vi "Multi_Run_Prog.vi"(0 "Command filename":path, 1 "Mode":T9(ring), 2 "Table":T6[](array[typedef]) {"Carrier_2 Q (l/min)" format="%#.2f"; "Row Duration (mins)" format="%#.1f"; "Row No" min=0; "Trace Gas Concentration (%)" min=0.0 format="%#_4f"; "Carrier_1 Q (l/min)" format="%#.2f"; "Tunnel Speed" format="%#.2f"; "Start X" format="%#.2f"; "Start Y" format="%#.2f"; "Start Z" format="%#.2f"; "End X" format="%#.2f"; "End Y" format="%#.2f"; "End Z" format="%#.2f"; "Averaging time (min)" min=0.0 format="%#.2f"}, 3 "Work in Tunnel Coordinates?":T1, 4 "Jump Bad Positions":bool) -> ()   [LabVIEW 2015]
uses:
  Anemometry Sub Vis/Gen Trav/Traverse_cluster.ctl
  Anemometry Sub Vis/Gen Trav/Spacing.ctl
  Anemometry Sub Vis/Controls/Multi_run_mode.ctl
  Anemometry Sub Vis/Gen Trav/Route mapping/Route_Display_Mode.ctl
  Anemometry Sub Vis/Controls/User_Specific_mode.ctl
  Anemometry Sub Vis/Controls/Multi_Run_Case.ctl
  Anemometry Sub Vis/Gen Trav/Multi_Run_Status.ctl
  Anemometry Sub Vis/Controls/Tunnel_Coordinates.ctl
  Anemometry Sub Vis/Controls/Post_Process.ctl
  ADAM Client/Sub VIs/ADAM Controls/Traverse_Level_State.ctl
  ADAM Client/Sub VIs/ADAM Controls/Tunnel_speed_mode.ctl
  Anemometry Sub Vis/Controls/Overhead.ctl
  ADAM Client/Sub VIs/ADAM Controls/Remember_value_mode.ctl
  Anemometry Sub Vis/Gen Trav/Trav_mode.ctl
  Anemometry Sub Vis/Controls/Home.ctl
  ADAM Client/Sub VIs/ADAM Controls/Client_Source_Status.ctl
  ADAM Client/Sub VIs/ADAM Controls/Update_scan_value.ctl
  Anemometry Sub Vis/File/Setup_Filetype.ctl
  Anemometry Sub Vis/Globals/Meas_global.vi
  Anemometry Sub Vis/Globals/Trav_pos_global.vi
  Anemometry Sub Vis/Globals/Preference_global.vi
  Anemometry Sub Vis/Gen Trav/Route mapping/Route_mapping_global.vi
  ADAM Serial/Instrument drivers/Traverses/~subVIs/DriveConfigGlobal.vi
  Anemometry Sub Vis/Globals/Extra_Commands_Global.vi
panel:
  in  "Sort Single\nMeasurements":bool
  out "Last Row Run":i32
  in  "Stop after Repeats":bool
  out "Current Overhead Factor":dbl format="%.3f"
  out "Estimated Completion time":string
  out "Max Tunnel Speed":dbl format="%.2f"
  out "Pause message":string
  in  "Pause":bool
  out "Non Starter":bool
  out "No of Rows":i32
  out "Status":T2
  in  "Synchronization Start No":i32=1 min=1 max=100
  out "Multi Run Case":T3
  out "Simulate/Run":T4
  in  "Display Mode":T5=enum."Display View on Crash"
  in  "stop":bool
  out "Currently on Row":i32
  # "X           Y            Z"
  # "Start"
  # "End"
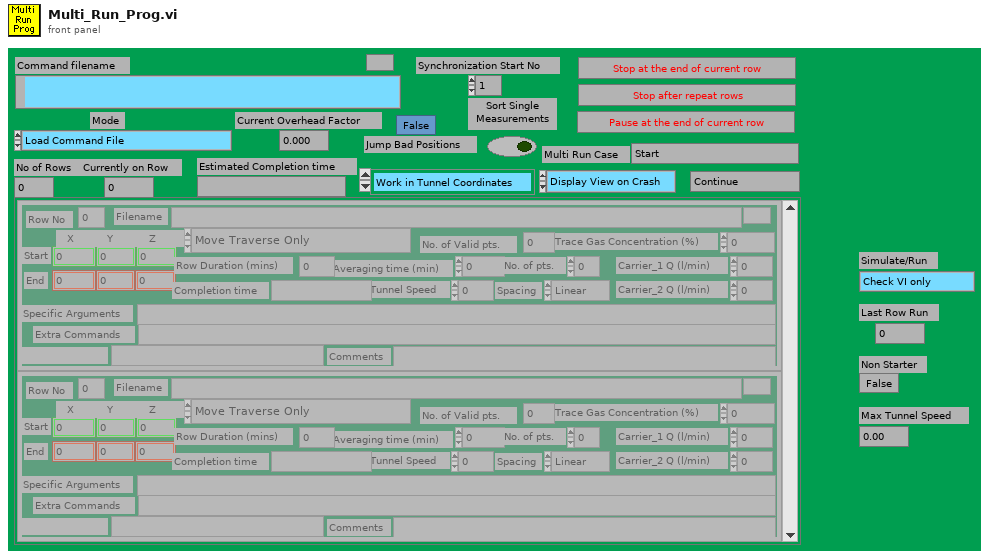
[diagram p1: front panel]
types:
  T1 = typedef "Tunnel_Coordinates.ctl" = enum16{"Work in Tunnel Coordinates", "Work in Model Coordinates"}
  T2 = typedef "Multi_Run_Status.ctl" = enum16{"Continue", "Jump to Next Point", "Jump to Next Row", "Jump To Fall Back", "Terminate Run"}
  T3 = typedef "Multi_Run_Case.ctl" = enum16{"Start", "Load Setup From File", "Has file been edited in Excel?", "Check Max Tunnel Speed", "Pre Check Row", "Check Rows", "Remove blank end rows", "Do results files already exist?", "FFID Bkgnd Measurements?", "First Save Setup file", "Setup Route checking", "Initialise Measurement Prog", "Input Current Position", "Experimental setup control", "Check source flowrates", "Setup for running mode", "Skip Blank Rows", "Which row to execute next", "Evaluate IF Statement", "Perform Measurement Setup", "Set Measurement Conditions", "Execute Row", "Calculate Row TIme", "Update time estimate", "Pause Multi Run Program", "Do Another Row?", "Find Next Fall Back Row", "Shut down source etc", "Email results to users", "Save run efficiency", "Remove Skipped Commands", "Show jumped positions", "Save Setup to File", "End"}
  T4 = typedef "User_Specific_mode.ctl" = enum16{"Check VI only", "Run VI"}
  T5 = typedef "Route_Display_Mode.ctl" = enum16{"Display View Always", "Display View on Crash"}
  T6 = typedef "Traverse_cluster.ctl" = cluster{"Start X":sgl, "Start Y":sgl, "Start Z":sgl, "End X":sgl, "End Y":sgl, "End Z":sgl, "No. of pts.":i32, "Spacing":T7, "Filename":path, "Tunnel Speed":dbl, "Averaging time (min)":dbl, "Extra Commands":string, "Carrier_1 Q (l/min)":dbl, "Carrier_2 Q (l/min)":dbl, "Trace Gas Concentration (%)":dbl, "Specific Arguments":string, "Comments":string, "Row No":i32, "Row Type Selector":T8, "Completion time":string, "Row Duration (mins)":dbl, "No. of Valid pts.":i32, "Meas Setup File":string}
  T7 = typedef "Spacing.ctl" = enum16{"Linear", "Log", "Gauss", "Specified", "N/A"}
  T8 = typedef "Multi_run_mode.ctl" = enum16{"Move Traverse Only", "Set Tunnel Speed Only", "Set Source Only", "Set Measurement Conditions", "Single Measurement", "Vertical Profile", "Lateral Profile", "Longitudinal Profile", "Explore Volume", "Multi-Axis Profile", "Auto Calibrate", "Meas Fast FID Bkgnd", "Check Beam Power", "Scanning Valve Measurement", "Run VI Named:", "Set ADAM Ch", "Wait (minutes)", "Send Message", "Synchronize With:", "Fall Back to this Row", "Turn Off Row Repeating", "Blank Row", "Traverse 3D Volume"}
  T9 = enum16{"Load Command File", "Save Command File", "Check Multi Run Prog", "Check Multi Run Prog With Live Moves", "Run Multi Run Prog"}
  T10 = typedef "Post_Process.ctl" = enum16{"Take New Data", "Post Process Raw Data File"}
  T11 = typedef "Traverse_Level_State.ctl" = enum16{"Running", "Complete"}
  T12 = enum32{"existing file", "new file", "new or existing file", "existing dir", "new dir", "new or existing dir", "existing file (use LLBs)", "new file (use LLBs)", "new or existing file (use LLBs)", "new or existing file or directory (use LLBs)"}
  T13 = typedef "Tunnel_speed_mode.ctl" = enum16{"Set Speed", "Set Speed then wait", "Is tunnel speed allowable?"}
  T14 = enum16{"All Channel Names", "Valid Channel Names"}
  T15 = typedef "Overhead.ctl" = enum16{"Update total times", "Read Current Overhead", "Re Scale totals to 3 hrs", "Initialise totals to 3hr"}
  T16 = typedef "Remember_value_mode.ctl" = enum16{"Read only", "Read and Write"}
  T17 = typedef "Home.ctl" = enum16{"Don't Home", "Home  +X", "Home  -X", "Home  +Y", "Home  -Y", "Home  +Z", "Home  -Z"}
  T18 = typedef "Trav_mode.ctl" = enum16{"Move traverse", "Read traverse position", "Teach Position"}
  T19 = typedef "Client_Source_Status.ctl" = enum16{"Not Using", "Using", "Must Have"}
  T20 = typedef "Update_scan_value.ctl" = cluster{"Channel Name":string, "New Value":dbl}
  T21 = typedef "Setup_Filetype.ctl" = enum16{"Measurement Setups", "Calibration Setups", "General", "Results File Plotter Setups", "Speed Calib Tweaks"}
  T22 = typedef "AxisConfigCluster.ctl" = cluster{"Channel Properties":T23, "Static Drive Configuration":T24}
  T23 = typedef "DriveProperties.ctl" = cluster{"Channel Name":string, "Vel. Default":sgl, "Acc. Default":sgl, "Vel. Max":sgl, "Vel. Min":sgl, "Acc. Max":sgl, "Acc. Min":sgl, "Pulses/unit":sgl, "Address":u8, "Pulse Offset":i32, "Pos Tolerance":sgl, "Pulses/rev":sgl, "Backlash/Eng units":sgl, "Current Pos":sgl, "Ch Status":enum16{"Active", "Offline", "Simulate"}, "Port Name":string, "Axis Transform mode":string, "Metadata Ch Name":string, "Type":string}
  T24 = typedef "DriveStaticConfig.ctl" = cluster{"Correction Gain % (CG)":u16, "Dead Band (DB)":i32, "Dead Band Window (DW)":i32, "Encoder Resolution (ER)":i32, "Step Mode  (FSB)":u16, "Position Maintenance (FSC)":u16, "Stop on Stall (FSD)":u16, "Activate OP1 on stall (FSE)":u16, "Stop on Trigger 3 (FSF)":u16, "OP2 in Deadband (FSG)":u16, "Stall Detect (FSH)":u16, "Limit Disable (LD)":u16, "Motor Resolution (MR)":enum16{"200", "400", "1000", "2000", "4000", "5000", "10000", "12800", "18000", "20000", "21600", "25000", "25400", "25600", "36000", "50000", "278528", "425984", "507904", "614400", "655360", "819200", "1024000"}, "Limit Switch Sense (OSA)":u16, "Home Position (OSB)":u16, "Home Switch Sense (OSC)":u16, "Encoder Z for Home (OSD)":u16, "Reference edge of Home (OSH)":u16, "RS232 Echo Control (SSA)":u16, "Buffer at Limit (SSG)":u16, "Buffer at Stop (SSH)":u16, "Indexer Mode  (FSA)":u16, "Type":string, "ConfigString":string, "De Power Motor":enum16{"TRUE", "FALSE"}}
  T25 = typedef "Status_Cluster.ctl" = cluster{"Status":T2, "Error Type":string, "Error Description":string}
  T26 = typedef "Server_Comms.ctl" = enum16{"Server Link Healthy", "Do Not Link To Server"}
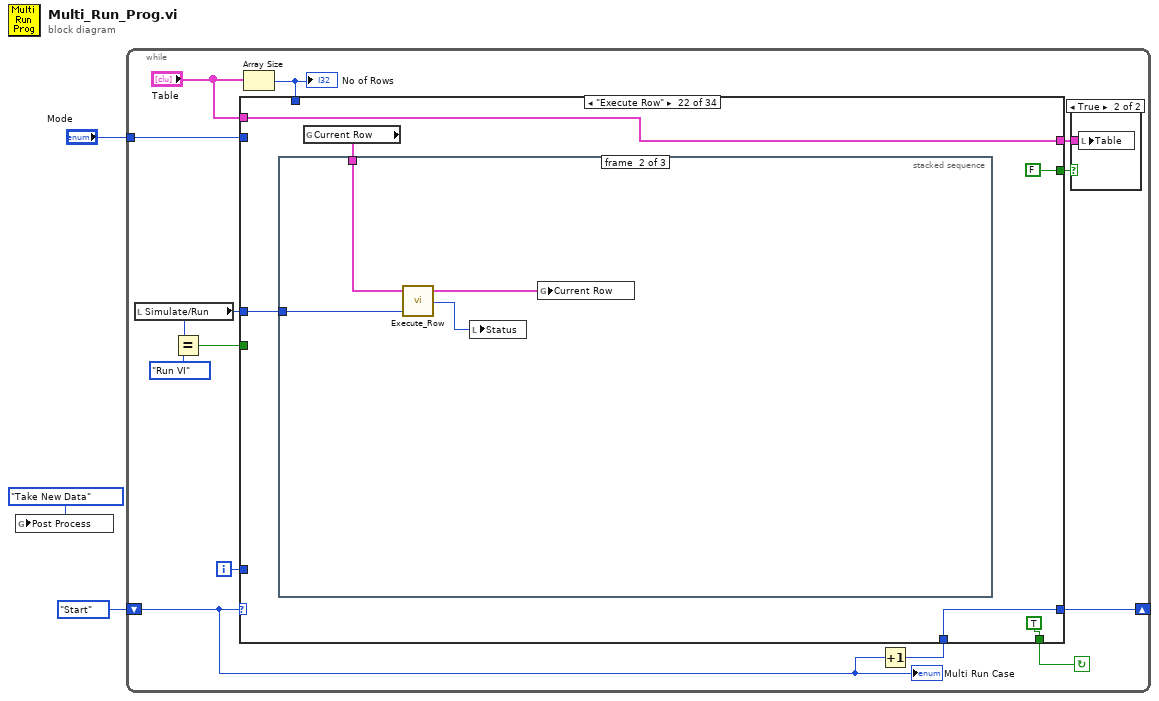
[diagram p0: block diagram]
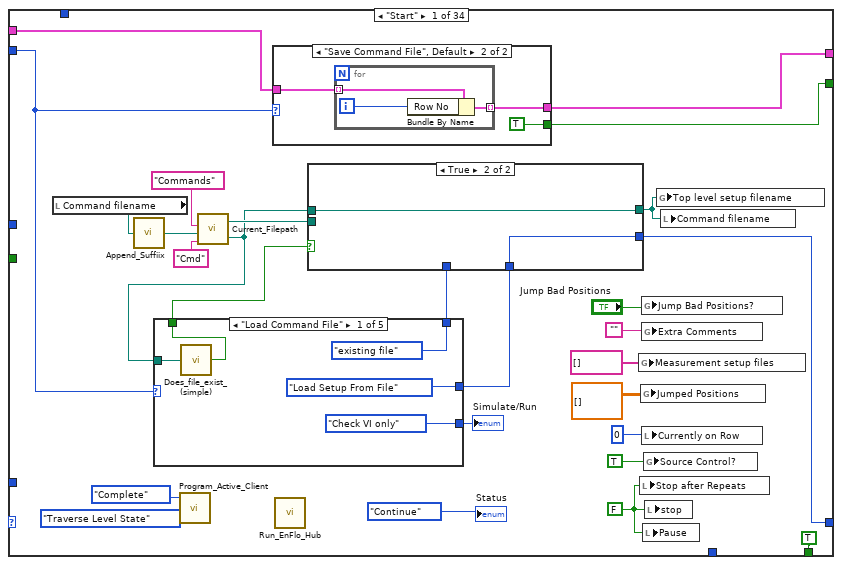
[diagram p3: hidden frame]
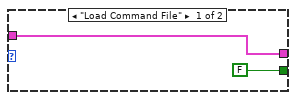
[diagram p4: hidden frame]
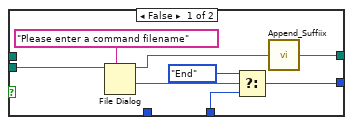
[diagram p5: hidden frame]
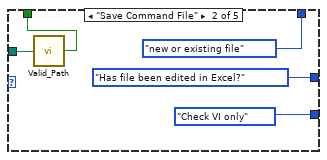
[diagram p6: hidden frame]
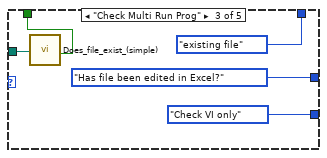
[diagram p7: hidden frame]
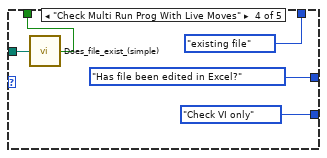
[diagram p8: hidden frame]
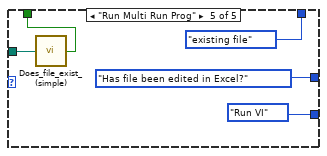
[diagram p9: hidden frame]
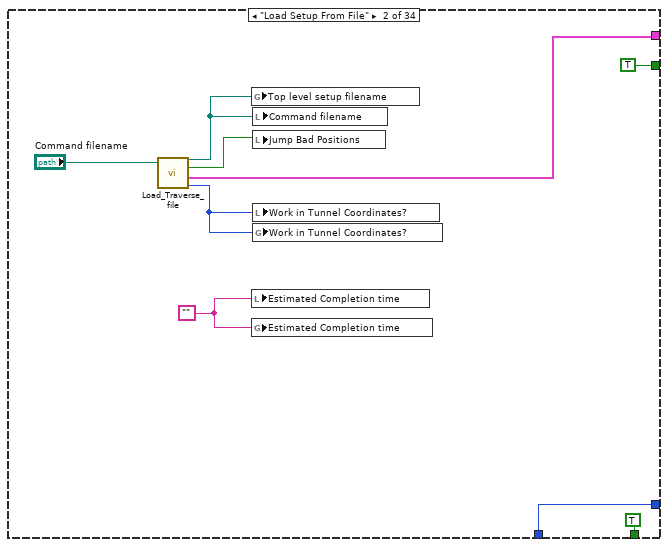
[diagram p10: hidden frame]
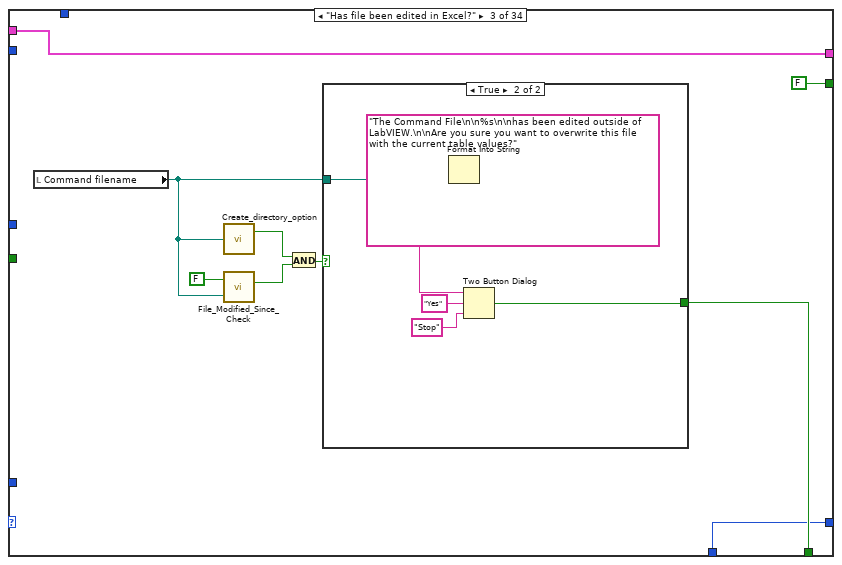
[diagram p11: hidden frame]
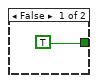
[diagram p12: hidden frame]
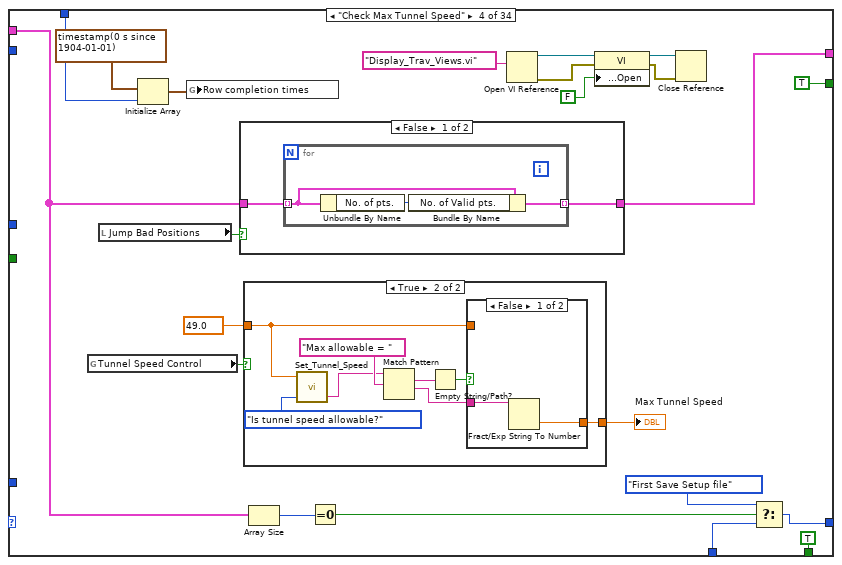
[diagram p13: hidden frame]
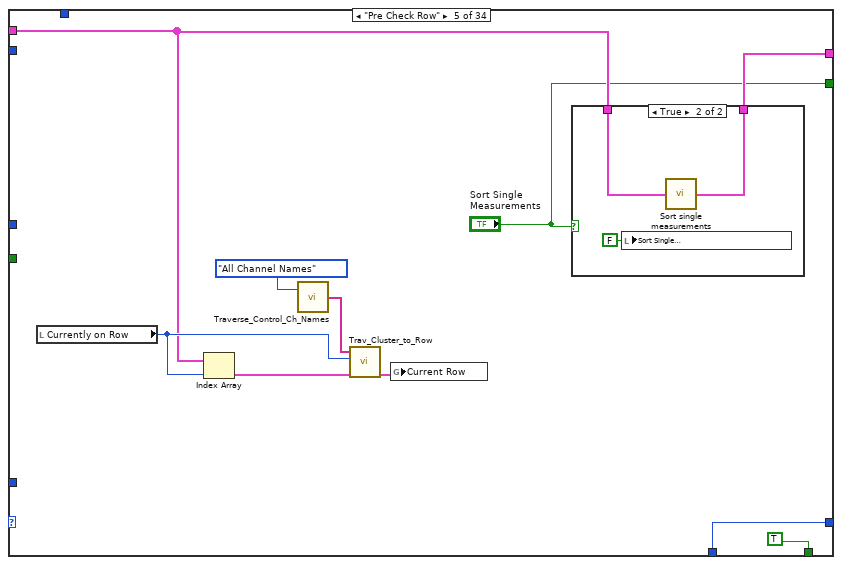
[diagram p17: hidden frame]
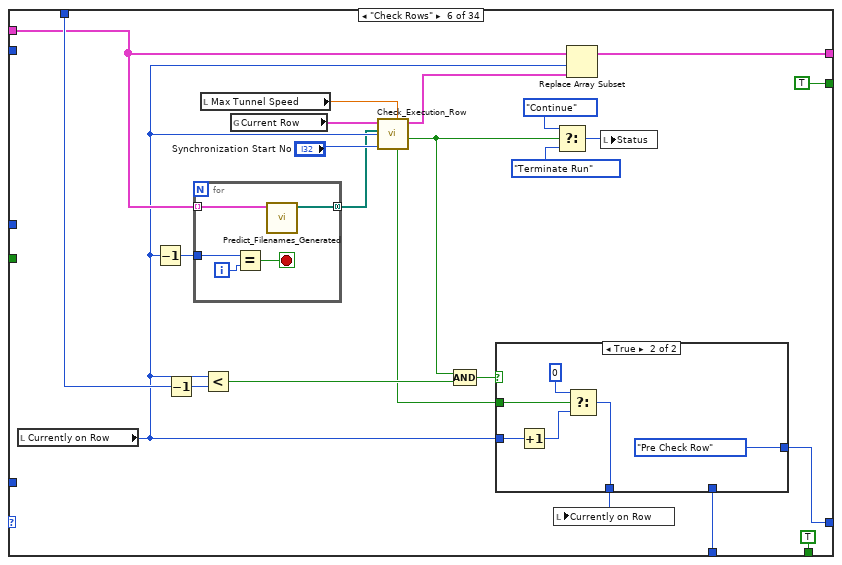
[diagram p19: hidden frame]
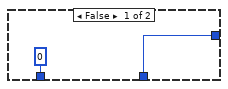
[diagram p20: hidden frame]
diagram:
  n1 = global write "Meas_global.vi" "Post Process"(Post_Process."Take New Data" ("Post Process")) -> ()
  n2 = while {
    shift-left: Multi_Run_Case."Start" ("Multi Run Case") -> [w12]
    shift-right: [w9] -> _
    tunnel: "Mode" -> [w15]
    i -> [w13]
    stop <- w16 continue-if-true
    n3 = local read "Simulate/Run"() -> (w5:T4)
    n4 = Equal?(x=w5, y=User_Specific_mode."Run VI" ("Simulate/Run")) -> (x = y?=w4:bool)
    n5 = Array Size(array="Table") -> (size(s)=w8:i32)
    "No of Rows" <- w8
    n6 = Increment(x=w12) -> (x+1=w14:T3)
    n7 = case shown="\"Execute Row\"" w12 {
      tunnel: [TRUE TRUE w100 TRUE TRUE TRUE TRUE TRUE TRUE TRUE TRUE ("Continue?") TRUE ("Continue?") TRUE TRUE TRUE w544 TRUE ("Continue?") TRUE ("Continue?") TRUE TRUE ("Continue?") TRUE TRUE TRUE TRUE TRUE TRUE TRUE TRUE TRUE TRUE TRUE TRUE TRUE FALSE] -> w16
      tunnel: w15 -> [w30 _ _ _ _ _ _ _ _ w426 _ _ _ _ _ _ _ _ _ _ _ _ _ _ _ _ _ _ _ _ _ _ w1267 _]
      tunnel: "Table" -> [w42 _ w97 w127 w155 w170 w204 w235 w393 w428 w451 w506 w518 w525 w533 w547 w609 w653 w757 w808 w820 w910 w944 w976 w1019 w1063 w1108 w1137 w1162 w1209 w1214 w1223 w1286 w1349]
      tunnel: w5 -> [_ _ _ _ _ _ _ w234 _ _ _ _ _ _ w532 w546 _ w651 _ w805 w817 w909 _ w973 _ w1069 _ _ _ _ _ _ w1277 _]
      tunnel: w14 -> [_ w93 w99 w125 w161 w176 w215 w238 w390 w425 w454 w504 w519 w524 w537 w549 w611 w649 w762 w809 w827 w907 w937 w978 w1022 _ _ w1123 w1164 w1211 w1217 w1231 w1284 w1348]
      tunnel: w13 -> [_ _ _ _ _ _ _ _ _ _ _ _ _ _ _ _ _ _ _ _ _ _ _ _ w1020 _ _ _ _ _ _ _ _ _]
      tunnel: [w40 w93 w99 w124 w161 w175 w215 w238 w390 w421 w454 w503 w519 w524 w535 w549 w611 w650 w761 w809 w828 w907 w937 w978 w1023 w1058 w1106 w1132 w1164 w1211 w1217 w1231 w1284 w1348] -> w9
      tunnel: [w29 TRUE FALSE ("Rows Added ?") TRUE ("Rows Added ?") "Sort Single\nMeasurements" TRUE TRUE FALSE FALSE TRUE FALSE FALSE FALSE FALSE FALSE TRUE FALSE ("Rows Added ?") FALSE ("Rows Added ?") FALSE FALSE ("Rows Added ?") FALSE FALSE FALSE TRUE ("Rows Added ?") FALSE FALSE FALSE FALSE FALSE FALSE TRUE TRUE TRUE FALSE] -> w10
      tunnel: w8 -> [_ _ _ w119 _ w180 w206 _ _ _ _ _ _ _ _ _ w612 w652 _ _ _ _ _ w972 _ w1061 w1099 _ _ _ _ _ w1258 _]
      tunnel: [w41 w94 w97 w129 w154 w183 w210 w235 w393 w429 w451 w506 w518 w525 w533 w545 w609 w654 w757 w808 w820 w910 w944 w975 w1019 w1063 w1108 w1137 w1162 w1209 w1213 w1223 w1285 w1349] -> w7
      tunnel: w4 -> [_ _ _ _ _ _ _ _ _ _ _ _ _ w522 w531 _ _ _ w751 _ _ _ w936 _ _ _ _ _ _ _ _ _ _ _]
      frame "Start" {
        w27 = FALSE ("Measurment setup Found?")
        n8 = local read "Command filename"() -> (w32:path)
        n9 = call "Append_Suffiix.vi"("Results file"=w32) -> ("appended path"=w22:path)
        n10 = call "Program_Active_Client.vi"("Mode"=enum16{"Program Active", "Traverse Level State"}."Traverse Level State", "Traverse level State"=Traverse_Level_State."Complete") -> ()  [unwired: 1 in, 3 out]
        n11 = call "Current_Filepath.vi"("Short_Name"="Cmd" ("Data Type"), "Filename in"=w22, "Data Type"="Commands") -> ("Filename Out"=w19:path, "Directory"=w21:path)  [unwired: 1 in]
        n12 = case shown="\"Load Command File\"" w30 {
          tunnel: [User_Specific_mode."Check VI only" ("Simulate/Run") User_Specific_mode."Check VI only" ("Simulate/Run") User_Specific_mode."Check VI only" ("Simulate/Run") User_Specific_mode."Check VI only" ("Simulate/Run") User_Specific_mode."Run VI" ("Simulate/Run")] -> w43
          tunnel: [Multi_Run_Case."Load Setup From File" ("Multi Run Case") Multi_Run_Case."Has file been edited in Excel?" ("Multi Run Case") Multi_Run_Case."Has file been edited in Excel?" ("Multi Run Case") Multi_Run_Case."Has file been edited in Excel?" ("Multi Run Case") Multi_Run_Case."Has file been edited in Excel?" ("Multi Run Case")] -> w39
          tunnel: [T12."existing file" ("select mode (2)") T12."new or existing file" ("select mode (2)") T12."existing file" ("select mode (2)") T12."existing file" ("select mode (2)") T12."existing file" ("select mode (2)")] -> w28
          tunnel: w19 -> [w64 w69 w73 w79 w84]
          tunnel: [w63 w68 w74 w78 w83] -> w18
          frame "Load Command File" {
            n13 = call "Does_file_exist_(simple).vi"("Pathname"=w64) -> ("exists?"=w63:bool)
          }
          frame "Save Command File" {
            n14 = call "Valid_Path.vi"("Filename"=w69) -> ("Valid Path?"=w68:bool)
          }
          frame "Check Multi Run Prog" {
            n15 = call "Does_file_exist_(simple).vi"("Pathname"=w73) -> ("exists?"=w74:bool)
          }
          frame "Check Multi Run Prog With Live Moves" {
            n16 = call "Does_file_exist_(simple).vi"("Pathname"=w79) -> ("exists?"=w78:bool)
          }
          frame "Run Multi Run Prog" {
            n17 = call "Does_file_exist_(simple).vi"("Pathname"=w84) -> ("exists?"=w83:bool)
          }
        }
        "Simulate/Run" <- w43
        n18 = case shown="\"Save Command File\", Default" w30 {
          tunnel: w42 -> [w46 w49]
          tunnel: [w46 w48] -> w41
          tunnel: [FALSE TRUE] -> w29
          frame "Load Command File" {
          }
          frame "Save Command File", Default {
            n19 = for {
              tunnel: w49 -> [w52] mode=indexing
              tunnel: [w51] -> w48 mode=indexing
              i -> [w50]
              n20 = Bundle By Name(cluster=w52, "Row No"=w50) -> (w51:T6)
            }
          }
        }
        n21 = call "Run_EnFlo_Hub.vi"() -> ()  [unwired: 8 out]
        n22 = case shown="True" w18 {
          tunnel: [w58 w62] -> w40
          tunnel: w39 -> [w59 w62]
          tunnel: w19 -> [_ w61]
          tunnel: [w57 w61] -> w31
          tunnel: w28 -> [_ _]
          tunnel: w21 -> [w53 _]
          frame False {
            n23 = File Dialog(7:"Please enter a command filename" ("prompt"), 11:w53) -> (1:w55:bool, 3:w56:path)  [unwired: 1 in, 6 out]
            n24 = Select(t=Multi_Run_Case."End" ("Multi Run Case"), s=w55, f=w59) -> (s? t:f=w58:T3)
            n25 = call "Append_Suffiix.vi"("Results file"=w56) -> ("appended path"=w57:path)
          }
          frame True {
          }
        }
        n26 = global write "Trav_pos_global.vi" "Measurement setup files"(string[] [] ("Measurement setup files")) -> ()
        n27 = local write "Stop after Repeats"(w27) -> ()
        n28 = global write "Trav_pos_global.vi" "Jumped Positions"(dbl[][] [] ("Jumped Positions")) -> ()
        n29 = global write "Trav_pos_global.vi" "Jump Bad Positions?"("Jump Bad Positions") -> ()
        n30 = global write "Meas_global.vi" "Extra Comments"("") -> ()
        n31 = local write "Currently on Row"(0 ("Currently on Row")) -> ()
        n32 = local write "Pause"(w27) -> ()
        n33 = global write "Trav_pos_global.vi" "Source Control?"(TRUE ("Source Control?")) -> ()
        n34 = local write "stop"(w27) -> ()
        n35 = global write "Trav_pos_global.vi" "Top level setup filename"(w31) -> ()
        n36 = local write "Command filename"(w31) -> ()
        "Status" <- Multi_Run_Status."Continue" ("Status")
      }
      frame "Load Setup From File" {
        w89 = ""
        n37 = call "Load_Traverse_file.vi"("Setup filename"="Command filename") -> ("Setup filename Out"=w91:path, "Jump Bad Positions"=w88:bool, "Table"=w94:T6[], "Work in Tunnel Coordinates?"=w90:T1)  [unwired: 2 out]
        n38 = global write "Trav_pos_global.vi" "Top level setup filename"(w91) -> ()
        n39 = local write "Estimated Completion time"(w89) -> ()
        n40 = global write "Trav_pos_global.vi" "Estimated Completion time"(w89) -> ()
        n41 = local write "Command filename"(w91) -> ()
        n42 = local write "Jump Bad Positions"(w88) -> ()
        n43 = local write "Work in Tunnel Coordinates?"(w90) -> ()
        n44 = global write "Trav_pos_global.vi" "Work in Tunnel Coordinates?"(w90) -> ()
      }
      frame "Has file been edited in Excel?" {
        n45 = local read "Command filename"() -> (w101:path)
        n46 = call "Create_directory_option.vi"("Filename"=w101) -> ("Path is to existing File"=w104:bool)  [unwired: 1 out]
        n47 = call "File_Modified_Since_Check.vi"("Pathname"=w101, "Just Modified?"=FALSE) -> ("Modified?"=w103:bool)
        n48 = And(x=w104, y=w103) -> (x .and. y?=w105:bool)
        n49 = case shown="True" w105 {
          tunnel: w101 -> [_ w112]
          tunnel: [TRUE ("T button?") w107] -> w100
          frame False {
          }
          frame True {
            n50 = Format Into String(format string="The Command File\n\n%s\n\nhas been edited outside of LabVIEW.\n\nAre you sure you want to overwrite this file  with the current table values?" ("Format String"), w112) -> (resulting string=w110:string)  [unwired: 2 in, 1 out]
            n51 = Two Button Dialog(message=w110, 1:"Stop" ("F button name (\"Cancel\")"), 2:"Yes" ("T button name (\"OK\")")) -> (T button?=w107:bool)
          }
        }
      }
      frame "Check Max Tunnel Speed" {
        n52 = global read "Preference_global.vi" "Tunnel Speed Control"() -> (w130:bool)
        n53 = local read "Jump Bad Positions"() -> (w128:bool)
        n54 = Initialize Array(timestamp(0 s since 1904-01-01) ("seconds since 1Jan1904"), w119) -> (w120:timestamp[])
        n55 = global write "Trav_pos_global.vi" "Row completion times"(w120) -> ()
        n56 = case shown="False" w128 {
          tunnel: w127 -> [w136 w140]
          tunnel: [w135 w140] -> w129
          frame False {
            n57 = for {
              tunnel: w136 -> [w138] mode=indexing
              tunnel: [w137] -> w135 mode=indexing
              n58 = Unbundle By Name(w138) -> ("No. of pts."=w139:i32)
              n59 = Bundle By Name(cluster=w138, "No. of Valid pts."=w139) -> (w137:T6)
            }
          }
          frame True {
          }
        }
        n60 = case shown="True" w130 {
          tunnel: 49.0 ("Tunnel Velocity m/s") -> [w141 w142]
          tunnel: [w141 w144] -> w132
          frame False {
          }
          frame True {
            n61 = call "Set_Tunnel_Speed.vi"("Mode"=Tunnel_speed_mode."Is tunnel speed allowable?", "Tunnel Velocity m/s"=w142) -> ("Error String"=w147:string)  [unwired: 1 in, 2 out]
            n62 = Match Pattern(string=w147, regular expression="Max allowable = ") -> (match substring=w146:string, after substring=w143:string)  [unwired: 3 out]
            n63 = Empty String/Path?(string/path=w146) -> (empty?=w145:bool)
            n64 = case shown="False" w145 {
              tunnel: [w150 w152] -> w144
              tunnel: w142 -> [_ w152]
              tunnel: w143 -> [w151 _]
              frame False {
                n65 = Fract/Exp String To Number(string=w151) -> (number=w150:dbl)  [unwired: 4 out]
              }
              frame True {
              }
            }
          }
        }
        "Max Tunnel Speed" <- w132
        n66 = Array Size(array=w127) -> (size(s)=w126:i32)
        n67 = Equal To 0?(x=w126) -> (x = 0?=w123:bool)
        n68 = Open VI Reference(vi path="Display_Trav_Views.vi" ("VI path")) -> (vi reference=w118:refnum<vi>, error out=w117:errorcluster)  [unwired: 1 in, 4 out]
        n69 = property class="VI"(reference=w118, error in=w117, "Front Panel Window:Open"=FALSE) -> (reference out=w115:refnum<vi>, error out=w114:errorcluster)
        n70 = Close Reference(reference=w115, error in (no error)=w114) -> ()  [unwired: 1 out]
        n71 = Select(t=Multi_Run_Case."First Save Setup file" ("Multi Run Case"), s=w123, f=w125) -> (s? t:f=w124:T3)
      }
      frame "Pre Check Row" {
        n72 = local read "Currently on Row"() -> (w158:i32)
        n73 = Index Array(array=w155, index=w158) -> (element=w159:T6)
        n74 = call "Traverse_Control_Ch_Names.vi"("Mode"=T14."All Channel Names") -> ("Channel names"=w156:string[])  [unwired: 1 in]
        n75 = call "Trav_Cluster_to_Row.vi"("Traverse line in"=w159, "Row Number"=w158, "Channel names"=w156) -> ("Traverse line Out"=w160:T6)  [unwired: 4 out]
        n76 = global write "Trav_pos_global.vi" "Current Row"(w160) -> ()
        n77 = case shown="True" "Sort Single\nMeasurements" {
          tunnel: w155 -> [w163 w166]
          tunnel: [w163 w165] -> w154
          frame False {
          }
          frame True {
            n78 = local write "Sort Single\nMeasurements"(FALSE ("Sort Single\nMeasurements")) -> ()
            n79 = call "Sort single measurements.vi"("Table In"=w166) -> ("Table Out"=w165:T6[])
          }
        }
      }
      frame "Check Rows" {
        n80 = local read "Currently on Row"() -> (w169:i32)
        n81 = Decrement(x=w169) -> (x-1=w168:i32)
        n82 = Decrement(x=w180) -> (x-1=w173:i32)
        n83 = for {
          tunnel: w170 -> [w194] mode=indexing
          tunnel: w168 -> [w192]
          tunnel: [w190] -> w167 mode=concatenating
          i -> [w193]
          stop <- w191 stop-if-true
          n84 = Equal?(x=w192, y=w193) -> (x = y?=w191:bool)
          n85 = call "Predict_Filenames_Generated.vi"("Traverse line"=w194) -> ("Filename"=w190:path[])  [unwired: 10 in]
        }
        n86 = local read "Max Tunnel Speed"() -> (w182:dbl)
        n87 = Less?(x=w169, y=w173) -> (x < y?=w179:bool)
        n88 = global read "Trav_pos_global.vi" "Current Row"() -> (w171:T6)
        n89 = call "Check_Execution_Row.vi"("Execution Row"=w171, "Earlier Filenames"=w167, "Synchronization Start No"="Synchronization Start No", "Row Index"=w169, "Max Tunnel Speed"=w182) -> ("Edited Row"=w172:bool, "Execution Row Out"=w174:T6, "Continue?"=w181:bool)  [unwired: 3 out]
        n90 = Compound Arithmetic op=AND(w181, w179) -> (w178:bool)
        n91 = case shown="True" w178 {
          tunnel: [0 w198] -> w177
          tunnel: w169 -> [_ w202]
          tunnel: w176 -> [w196 _]
          tunnel: [w196 Multi_Run_Case."Pre Check Row" ("Multi Run Case")] -> w175
          tunnel: w172 -> [_ w200]
          frame False {
          }
          frame True {
            n92 = Increment(x=w202) -> (x+1=w199:i32)
            n93 = Select(t=0, s=w200, f=w199) -> (s? t:f=w198:i32)
          }
        }
        n94 = local write "Currently on Row"(w177) -> ()
        n95 = Select(t=Multi_Run_Status."Continue" ("Status"), s=w181, f=Multi_Run_Status."Terminate Run" ("Status")) -> (s? t:f=w187:T2)
        n96 = Replace Array Subset(array=w170, new element=w174, index=w169) -> (w183:T6[])
        n97 = local write "Status"(w187) -> ()
      }
      frame "Remove blank end rows" {
        n98 = local read "Jump Bad Positions"() -> (w203:bool)
        n99 = case shown="False" w203 {
          tunnel: w206 -> [w221 _]
          tunnel: w204 -> [w220 w224]
          tunnel: [w218 w224] -> w205
          frame False {
            n100 = call "Calc_Remaining_Time.vi"("Currently on Row"=-1 ("Start Index"), "Table In"=w220) -> ("Table Out"=w218:T6[])  [unwired: 1 out]
            n101 = Decrement(x=w221) -> (x-1=w223:i32)
            n102 = Index Array(array=w218, index=w223) -> (element=w222:T6)
            n103 = Unbundle By Name(w222) -> ("Completion time"=w217:string)
            n104 = global write "Trav_pos_global.vi" "Estimated Completion time"(w217) -> ()
            n105 = local write "Estimated Completion time"(w217) -> ()
          }
          frame True {
          }
        }
        n106 = Reverse 1D Array(array=w205) -> (reversed array=w214:T6[])
        n107 = while {
          tunnel: [w225] -> w212
          tunnel: w206 -> [w229]
          tunnel: w214 -> [w233] mode=indexing
          i -> [w225]
          stop <- w226 continue-if-true
          n108 = Unbundle By Name(w233) -> ("Row Type Selector"=w231:T8)
          n109 = Increment(x=w225) -> (x+1=w230:i32)
          n110 = Greater?(x=w229, y=w230) -> (0:w228:bool)
          n111 = Equal?(x=Multi_run_mode."Blank Row" ("Row Type Selector"), y=w231) -> (x = y?=w227:bool)
          n112 = And(x=w227, y=w228) -> (x .and. y?=w226:bool)
        }
        n113 = Subtract(x=w206, y=w212) -> (x-y=w211:i32)
        n114 = call "Overhead_Factor.vi"("Mode"=Overhead."Read Current Overhead") -> ("Current Overhead Factor"=w207:dbl)  [unwired: 3 in]
        n115 = local write "Current Overhead Factor"(w207) -> ()
        n116 = Array Subset(array=w205, index=0 ("Array Index"), length=w211) -> (w210:T6[])
      }
      frame "Do results files already exist?" {
        n117 = for {
          tunnel: w235 -> [w247] mode=indexing
          shift-right: [w243] -> _
          shift-left: path[] [] -> [w244]
          tunnel: w234 -> [w241]
          n118 = Unbundle By Name(w247) -> ("Specific Arguments"=w240:string, "Row Type Selector"=w246:T8, "Filename"=w245:path)
          n119 = while {
            shift-left: w244 -> [w255]
            shift-right: [w254] -> w243
            tunnel: w245 -> [w256]
            tunnel: w246 -> [w260]
            shift-left: 0 -> [w261]
            shift-right: [w257] -> _
            tunnel: w241 -> [w251]
            shift-right: [w250] -> _
            shift-left: _ -> [w249]
            tunnel: w240 -> [w248]
            stop <- w259 continue-if-true
            n120 = Increment(x=w261) -> (x+1=w258:i32)
            n121 = case shown="0, Default" w261 {
              tunnel: w260 -> [w270 _ _ _ _ _ _ _ _ _ _ _]
              tunnel: [w265 w292 w297 w304 w309 TRUE ("exists?") TRUE ("exists?") FALSE ("exists?") FALSE ("exists?") TRUE ("true") w366 w379] -> w259
              tunnel: w258 -> [w272 w295 w300 w303 w310 w315 w326 w337 w348 w352 w364 _]
              tunnel: [w272 w295 w300 w303 w310 w313 w325 w337 w348 w353 w364 w378] -> w257
              tunnel: [w271 w294 w299 w302 w307 w323 w334 w339 w341 w350 w368 w384] -> w254
              tunnel: w255 -> [w271 w294 w299 w302 w308 w323 w334 w339 w341 w350 w368 w384]
              tunnel: w256 -> [w264 _ _ _ _ _ _ _ _ _ _ _]
              tunnel: 7 -> [_ _ _ _ _ _ _ _ _ w351 _ w378]
              tunnel: 9 -> [_ _ _ _ _ w314 _ _ _ _ _ _]
              tunnel: w251 -> [_ _ _ _ _ _ _ _ _ _ w367 _]
              tunnel: [w263 w291 w296 w301 w306 w311 w324 w335 w340 w349 w365 w377] -> w250
              tunnel: w249 -> [_ w291 w296 w301 w306 w311 w324 w335 w340 w349 w365 w377]
              tunnel: w248 -> [w262 _ _ _ _ _ _ _ _ _ _ _]
              frame 0, Default {
                n122 = case shown="\"Run VI Named:\"" w270 {
                  tunnel: [TRUE w283 FALSE FALSE] -> w267
                  tunnel: w264 -> [w273 w282 w287 w289]
                  tunnel: w262 -> [_ w280 _ _]
                  tunnel: [w273 w282 w287 w289] -> w263
                  frame "Move Traverse Only", Default {
                  }
                  frame "Run VI Named:" {
                    n123 = Match Pattern(string=w280, regular expression=";") -> (before substring=w279:string)  [unwired: 4 out]
                    n124 = call <vilib>:"Trim Whitespace.vi"("string"=w279) -> ("trimmed string"=w277:string)  [unwired: 1 in]
                    n125 = Equal?(x=w277, y="Pressure_Tapped_Cube.vi") -> (x = y?=w284:bool)
                    n126 = Equal?(x=w277, y="Take_Data_on_the_Move.vi") -> (x = y?=w278:bool)
                    n127 = Equal?(x=w277, y="Capture_Flow_Vis.vi") -> (x = y?=w275:bool)
                    n128 = Compound Arithmetic op=OR(w284, w278, w275) -> (w283:bool)
                  }
                  frame "Auto Calibrate" {
                  }
                  frame "Send Message" {
                  }
                }
                n129 = local read "Status"() -> (w268:T2)
                n130 = Not Equal?(x=Multi_Run_Status."Terminate Run" ("Status"), y=w268) -> (x != y?=w266:bool)
                n131 = And(x=w267, y=w266) -> (x .and. y?=w265:bool)
              }
              frame 1 {
                n132 = Not Equal?(x=path "", y=w291) -> (x != y?=w292:bool)
              }
              frame 2 {
                n133 = Not Equal?(x=w296, y=path "") -> (x != y?=w297:bool)
              }
              frame 3 {
                n134 = Search 1D Array(1D array=w302, element=w301) -> (index of element=w305:i32)  [unwired: 1 out]
                n135 = Less Than 0?(x=w305) -> (x < 0?=w304:bool)
              }
              frame 4 {
                n136 = Build Array (concatenate)(w308, w306) -> (w307:path[])
                n137 = call "Does_file_exist_(simple).vi"("Pathname"=w306) -> ("exists?"=w309:bool)
              }
              frame 5 {
                n138 = Path To String(path=w311) -> (string=w322:string)
                n139 = global read "Meas_global.vi" "Start Time of experiment"() -> (w317:dbl)
                n140 = Concatenate Strings(w322, "Append" ("Substring")) -> (w320:string)
                n141 = call "Remember_value.vi"("Mode"=Remember_value_mode."Read only", "Ch name"=w320) -> ("Output Value"=w318:dbl)  [unwired: 1 in]
                n142 = Not Equal?(x=w317, y=w318) -> (x != y?=w316:bool)
                n143 = Select(t=w315, s=w316, f=w314) -> (s? t:f=w313:i32)
              }
              frame 6 {
                n144 = Increment(x=w326) -> (x+1=w327:i32)
                n145 = Format Into String(format string="The results filename \"%s\" already exists.\nDo you wish to append to this file during the run?" ("Format String"), w324) -> (resulting string=w331:string)  [unwired: 2 in, 1 out]
                n146 = Two Button Dialog(message=w331, 1:"Abort Run" ("F button name (\"Cancel\")"), 2:"Append" ("T button name (\"OK\")")) -> (T button?=w328:bool)
                n147 = Select(t=w327, s=w328, f=w326) -> (s? t:f=w325:i32)
              }
              frame 7 {
                n148 = local write "Status"(Multi_Run_Status."Terminate Run" ("Status")) -> ()
              }
              frame 8 {
                n149 = Path To String(path=w340) -> (string=w347:string)
                n150 = Concatenate Strings(w347, "Append" ("Substring")) -> (w345:string)
                n151 = global read "Meas_global.vi" "Start Time of experiment"() -> (w342:dbl)
                n152 = call "Remember_value.vi"("Mode"=Remember_value_mode."Read and Write", "Input Value"=w342, "Ch name"=w345) -> ()  [unwired: 1 out]
              }
              frame 9 {
                n153 = call "Read_File_Simple.vi"("Filename"=w349) -> ("string"=w356:string)  [unwired: 2 in, 7 out]
                n154 = call "Is_it_a_Results_File.vi"("character string"=w356) -> ("Results File?"=w355:bool)  [unwired: 2 out]
                n155 = case shown="False" w355 {
                  tunnel: w349 -> [w359 _]
                  tunnel: [w357 w363] -> w353
                  tunnel: w352 -> [_ w363]
                  tunnel: w351 -> [w357 _]
                  frame False {
                    n156 = Path To String(path=w359) -> (string=w361:string)
                    n157 = Format Into String(format string="The File %s is not in the correct Results file format.\nCheck that it is tab delimited rather than excel format, or choose another file." ("Format String"), w361) -> (resulting string=w358:string)  [unwired: 2 in, 1 out]
                    n158 = One Button Dialog(message=w358, button name ("OK")="Stop") -> ()  [unwired: 1 out]
                  }
                  frame True {
                  }
                }
              }
              frame 10 {
                n159 = case shown="\"Run VI\"" w367 {
                  tunnel: w365 -> [_ w376]
                  tunnel: [FALSE ("exists?") w370] -> w366
                  frame "Check VI only", Default {
                  }
                  frame "Run VI" {
                    n160 = call "Open_File_for_write.vi"("append to file? (new file:F)"=TRUE, "file path"=w376) -> ("error out"=w374:errorcluster, "refnum"=w375:refnum<file>)  [unwired: 1 in, 7 out]
                    n161 = Unbundle By Name(w374) -> ("code"=w373:i32)
                    n162 = Close File(refnum=w375, error in=w374) -> ()  [unwired: 2 out]
                    n163 = Equal?(x=10 ("code"), y=w373) -> (x = y?=w370:bool)
                  }
                }
              }
              frame 11 {
                n164 = Path To String(path=w377) -> (string=w382:string)
                n165 = Format Into String(format string="The File %s is already open in another application." ("Format String"), w382) -> (resulting string=w381:string)  [unwired: 2 in, 1 out]
                n166 = One Button Dialog(message=w381, button name ("OK")="Stop") -> (true=w379:bool)
              }
            }
          }
        }
      }
      frame "FFID Bkgnd Measurements?" {
        n167 = for {
          tunnel: w393 -> [w406] mode=indexing
          tunnel: [w404] -> w392 mode=indexing
          tunnel: [w403] -> w391 mode=indexing
          tunnel: [w401] -> w386 mode=indexing
          n168 = Unbundle By Name(w406) -> ("Specific Arguments"=w402:string, "Carrier_1 Q (l/min)"=w399:dbl, "Carrier_2 Q (l/min)"=w398:dbl, "Row Type Selector"=w400:T8)
          n169 = Add(x=w399, y=w398) -> (x+y=w397:dbl)
          n170 = case shown="\"Auto Calibrate\"" w400 {
            tunnel: w397 -> [w409 _]
            tunnel: [FALSE w410] -> w403
            tunnel: w402 -> [_ w411]
            tunnel: [w408 w410] -> w401
            frame Default {
              n171 = Greater Than 0?(x=w409) -> (x > 0?=w408:bool)
            }
            frame "Auto Calibrate" {
              n172 = call "Get_array_values_fr_String.vi"("String Value"=w411) -> ("String array"=w414:string[])  [unwired: 1 out]
              n173 = Index Array(array=w414, index=0 ("Index")) -> (element=w413:string)
              n174 = Equal?(x=w413, y="Concentration") -> (x = y?=w410:bool)
            }
          }
          n175 = Equal?(x=Multi_run_mode."Meas Fast FID Bkgnd" ("Row Type Selector"), y=w400) -> (x = y?=w404:bool)
        }
        n176 = Or Array Elements(Boolean array=w392) -> (logical OR=w388:bool)
        n177 = Or Array Elements(Boolean array=w386) -> (logical OR=w385:bool)
        n178 = Or Array Elements(Boolean array=w391) -> (logical OR=w387:bool)
        n179 = global write "Trav_pos_global.vi" "Source Control?"(w385) -> ()
        n180 = Compound Arithmetic op=AND(w387, invert w388) -> (w389:bool)
        n181 = case shown="True" w389 {
          frame False {
          }
          frame True {
            n182 = One Button Dialog(message="This run automatically calibrates the Fast FID but does not have a Meas Fast FID Bkgnd row" ("format string")) -> ()  [unwired: 2 out]
          }
        }
      }
      frame "First Save Setup file" {
        w416 = -1 ("Currently on Row")
        n183 = global write "Trav_pos_global.vi" "Work in Tunnel Coordinates?"("Work in Tunnel Coordinates?") -> ()
        n184 = case shown="\"Save Command File\"" w426 {
          tunnel: [w433 w435 w437 Multi_Run_Case."End" ("Multi Run Case") Multi_Run_Case."End" ("Multi Run Case")] -> w420
          tunnel: w425 -> [w433 w435 w437 _ _]
          tunnel: [w434 w436 w438 w439 w441] -> w419
          frame "Run Multi Run Prog" {
            w434 = FALSE  # Live Traverse Preview?
          }
          frame "Check Multi Run Prog With Live Moves" {
            w436 = TRUE  # Live Traverse Preview?
          }
          frame "Check Multi Run Prog" {
            w438 = FALSE  # Live Traverse Preview?
          }
          frame "Load Command File" {
            w439 = FALSE  # Live Traverse Preview?
          }
          frame "Save Command File" {
            w441 = FALSE  # Live Traverse Preview?
          }
        }
        n185 = local read "Command filename"() -> (w427:path)
        n186 = local read "Jump Bad Positions"() -> (w417:bool)
        n187 = call "Save_Trav_setup.vi"("Work in Tunnel Coordinates?"="Work in Tunnel Coordinates?", "Trav Table"=w428, "Jump Bad Positions"=w417, "Setup filename"=w427) -> ("Trav Table Out"=w429:T6[])  [unwired: 1 out]
        n188 = local read "Status"() -> (w422:T2)
        n189 = global write "Meas_global.vi" "Extra Comments"("") -> ()
        n190 = local write "Currently on Row"(w416) -> ()
        n191 = local write "Last Row Run"(w416) -> ()
        n192 = case shown="\"Continue\"" w422 {
          tunnel: [w431 Multi_Run_Case."End" ("Multi Run Case")] -> w421
          tunnel: w420 -> [w431 _]
          frame "Continue" {
          }
          frame "Jump to Next Point", Default {
          }
        }
        n193 = global write "Trav_pos_global.vi" "Live Traverse Preview?"(w419) -> ()
      }
      frame "Setup Route checking" {
        w447 = string[] []
        n194 = global read "Trav_pos_global.vi" "Work in Tunnel Coordinates?"() -> (w448:T1)
        n195 = for {
          tunnel: w451 -> [w492] mode=indexing
          shift-right: [w483] -> w449
          shift-left: string[] [] -> [w484]
          n196 = Unbundle By Name(w492) -> ("Extra Commands"=w485:string, "Start X"=w489:sgl, "Start Y"=w488:sgl, "Start Z"=w487:sgl)
          n197 = Build Array(w489, w488, w487) -> (w490:sgl[])
          n198 = Not A Number/Path/Refnum?(number/path/refnum=w490) -> (NaN/Path/Refnum?=w491:bool[])
          n199 = Or Array Elements(Boolean array=w491) -> (logical OR=w486:bool)
          n200 = case shown="False" w486 {
            tunnel: w485 -> [w496 _]
            tunnel: w484 -> [w495 w497]
            tunnel: [w494 w497] -> w483
            frame False {
              n201 = call "Which_Trav_Setup.vi"("Extra Command String"=w496) -> ("Traverse Setups"=w493:string[])
              n202 = Build Array (concatenate)(w495, w493) -> (w494:string[])
            }
            frame True {
            }
          }
        }
        n203 = call "Analyse_string_array.vi"("String array"=w449) -> ("Unique strings"=w444:string[])  [unwired: 2 out]
        n204 = for {
          tunnel: w444 -> [w460] mode=indexing
          tunnel: w448 -> [w459]
          shift-right: [w458] -> w445
          shift-left: w447 -> [w457]
          shift-right: [w455] -> w446
          shift-left: w447 -> [w456]
          n205 = stacked-sequence {
            tunnel: w460 -> [w466 w471]
            tunnel: w459 -> [w463 _]
            tunnel: [_ w470] -> w458
            tunnel: w457 -> [_ w469]
            tunnel: w456 -> [_ w468]
            tunnel: [_ w467] -> w455
            frame #0 {
              w461 = TRUE  # Last Part of Move?
              n206 = call "3D_Traverse_move.vi"("Mode"=Trav_mode."Read traverse position", "Work in Tunnel Coordinates"=w463, "Home"=Home."Don't Home", "Simulate/Run"=User_Specific_mode."Run VI", "Traverse name"=w466, "Last Part of Move?"=w461) -> ()  [unwired: 11 in, 3 out]
            }
            frame #1 {
              n207 = global read "DriveConfigGlobal.vi" "Configurations"() -> (w472:T22[])
              n208 = for {
                tunnel: w472 -> [w482] mode=indexing
                tunnel: w471 -> [w479]
                shift-right: [w477] -> w470
                shift-left: w469 -> [w478]
                shift-right: [w473] -> w467
                shift-left: w468 -> [w474]
                i -> [w481]
                n209 = Unbundle By Name(w482) -> ("Channel Properties.Metadata Ch Name"=w476:string)
                n210 = Format Into String(format string="%d", initial string=w479, w481) -> (resulting string=w475:string)  [unwired: 1 in, 1 out]
                n211 = Build Array (concatenate)(w478, w476) -> (w477:string[])
                n212 = Build Array (concatenate)(w474, w475) -> (w473:string[])
              }
            }
          }
        }
        n213 = global write "Trav_pos_global.vi" "Traverses to Move"(w444) -> ()
        n214 = global write "Trav_pos_global.vi" "ADAM Positions Ch names"(w445) -> ()
        n215 = global write "Route_mapping_global.vi" "Display Mode"("Display Mode") -> ()
        n216 = global write "Trav_pos_global.vi" "Route checking Chs"(w446) -> ()
      }
      frame "Initialise Measurement Prog" {
        n217 = for {
          tunnel: w506 -> [w517] mode=indexing
          tunnel: [w515] -> w500 mode=concatenating
          n218 = Unbundle By Name(w517) -> ("Meas Setup File"=w516:string)
          n219 = call "Get_array_values_fr_String.vi"("String Value"=w516) -> ("String array"=w515:string[])  [unwired: 1 out]
        }
        n220 = call "Analyse_string_array.vi"("String array"=w500) -> ("Unique strings"=w499:string[])  [unwired: 1 in, 1 out]
        n221 = for {
          tunnel: w499 -> [w510] mode=indexing
          tunnel: [w510] -> w498 mode=indexing if=w509
          n222 = String Subset(string=w510, offset (0)=2, length (rest)=4 ("length (rest)")) -> (substring=w512:string)
          n223 = Not Equal?(x=w512, y="----" ("f")) -> (x != y?=w509:bool)
        }
        n224 = call "Perform_Meas_Setup.vi"("Simulate/Run"=User_Specific_mode."Check VI only", "String array"=w498) -> ("Continue?"=w501:bool)  [unwired: 1 out]
        n225 = Select(t=w504, s=w501, f=Multi_Run_Case."End" ("Multi Run Case")) -> (s? t:f=w503:T3)
      }
      frame "Input Current Position" {
        n226 = call "Save_ADAM_Table_Locally.vi"() -> ()  [unwired: 12 in]
      }
      frame "Experimental setup control" {
        # "#Check- Should this be AND?"
        n227 = global read "Trav_pos_global.vi" "Source Control?"() -> (w526:bool)
        n228 = Or(x=w526, y=w522) -> (x .or. y?=w527:bool)
        n229 = case shown="True" w527 {
          tunnel: w526 -> [_ w530]
          frame False {
          }
          frame True {
            n230 = call "Exp_Setup_Control.vi"("Dispersion?"=w530) -> ()  [unwired: 3 out]
          }
        }
        n231 = global write "Trav_pos_global.vi" "FFID Background"(T6 {"Start X"=0.0, "Start Y"=0.0, "Start Z"=0.0, "End X"=0.0, "End Y"=0.0, "End Z"=0.0, "No. of pts."=0, "Spacing"=enum."Linear", "Filename"=path "", "Tunnel Speed"=0.0, "Averaging time (min)"=0.0, "Extra Commands"="", "Carrier_1 Q (l/min)"=0.0, "Carrier_2 Q (l/min)"=0.0, "Trace Gas Concentration (%)"=0.0, "Specific Arguments"="", "Comments"="", "Row No"=0, "Row Type Selector"=enum."Move Traverse Only", "Completion time"="", "Row Duration (mins)"=0.0, "No. of Valid pts."=0, "Meas Setup File"=""} ("FFID Background")) -> ()
      }
      frame "Check source flowrates" {
        # "#Check- shouldn't we check source flowrates in \"Check\" mode too...?"
        n232 = case shown="\"Run VI\"" w532 {
          tunnel: w533 -> [_ w540]
          frame "Check VI only", Default {
            n233 = Get Date/Time In Seconds() -> (seconds since 1Jan1904=w539:timestamp)
            n234 = global write "Trav_pos_global.vi" "Simulation Time"(w539) -> ()
          }
          frame "Run VI" {
            n235 = for {
              tunnel: w540 -> [w541] mode=indexing
              n236 = call "Set_Source.vi"("Source Status"=Client_Source_Status."Using", "Traverse line"=w541, "Simulate/Run"=User_Specific_mode."Check VI only") -> ()  [unwired: 1 in, 6 out]
            }
          }
        }
        n237 = Increment(x=w537) -> (x+1=w534:T3)
        n238 = Select(t=w537, s=w531, f=w534) -> (s? t:f=w535:T3)
      }
      frame "Setup for running mode" {
        n239 = stacked-sequence {
          seq-local: [_ _ _ _ _ w588 _] -> [_ _ _ _ _ _ w605]
          seq-local: [_ _ _ _ w577 _ _] -> [_ _ _ _ _ w587 _]
          tunnel: w547 -> [w552 _ _ w576 w579 _ _]
          tunnel: w546 -> [_ _ w571 _ _ _ _]
          tunnel: [_ _ _ w574 _ _ _] -> w545
          tunnel: [_ _ _ _ _ w588 _] -> w544
          frame #0 {
            n240 = for {
              tunnel: w552 -> [w556] mode=indexing
              tunnel: [w553] -> w551 mode=indexing
              n241 = Unbundle By Name(w556) -> ("Row Type Selector"=w555:T8)
              n242 = Equal?(x=Multi_run_mode."Synchronize With:" ("Row Type Selector"), y=w555) -> (x = y?=w553:bool)
            }
            n243 = call "Setup_Environment.vi"() -> ()  [unwired: 1 in, 1 out]
            n244 = Or Array Elements(Boolean array=w551) -> (logical OR=w550:bool)
            n245 = case shown="True" w550 {
              frame False {
              }
              frame True {
                n246 = call "Declare_Sync_Client.vi"() -> ()  [unwired: 6 out]
              }
            }
          }
          frame #1 {
            n247 = Open VI Reference(vi path="Display_Trav_Views.vi" ("VI path")) -> (vi reference=w562:refnum<vi>, error out=w561:errorcluster)  [unwired: 1 in, 4 out]
            n248 = global write "Meas_global.vi" "Post Process"(Post_Process."Take New Data" ("Post Process")) -> ()
            n249 = property class="VI"(reference=w562, error in=w561, "Front Panel Window:Open"=FALSE) -> (reference out=w559:refnum<vi>, error out=w558:errorcluster)
            n250 = Close Reference(reference=w559, error in (no error)=w558) -> ()  [unwired: 1 out]
          }
          frame #2 {
            w566 = TRUE  # Start of Multi Run Prog
            w572 = TRUE
            n251 = Get Date/Time In Seconds() -> (seconds since 1Jan1904=w565:timestamp)
            n252 = local read "Command filename"() -> (w570:path)
            n253 = To Double Precision Float(number=w565) -> (double precision float=w564:dbl)
            n254 = global write "Preference_global.vi" "Unblock Email"(w572) -> ()
            n255 = global write "Meas_global.vi" "Start Time of experiment"(w564) -> ()
            n256 = global write "Preference_global.vi" "Unblock SMS"(w572) -> ()
            n257 = Path To String(path=w570) -> (string=w568:string)
            n258 = Concatenate Strings("Commencing a new multi run Prog having the setup filename of :" ("Message"), w568) -> (w567:string)
            n259 = call "Log_Current_row_to_Execute.vi"("Simulate/Run"=w571, "Message"=w567, "Start of Multi Run Prog"=w566) -> ()  [unwired: 2 in, 5 out]
          }
          frame #3 {
            n260 = call "Calc_Remaining_Time.vi"("Currently on Row"=-1, "Table In"=w576) -> ("Estimated Completion time"=w573:string, "Table Out"=w574:T6[])
            n261 = local write "Estimated Completion time"(w573) -> ()
            n262 = global write "Trav_pos_global.vi" "Estimated Completion time"(w573) -> ()
          }
          frame #4 {
            n263 = global read "Trav_pos_global.vi" "Source Control?"() -> (w578:bool)
            n264 = case shown="True" w578 {
              tunnel: w579 -> [_ w583]
              tunnel: [FALSE w581] -> w577
              frame False {
              }
              frame True {
                n265 = for {
                  tunnel: w583 -> [w586] mode=indexing
                  tunnel: [w584] -> w582 mode=indexing
                  n266 = Unbundle By Name(w586) -> ("Trace Gas Concentration (%)"=w585:dbl)
                  n267 = Greater Than 0?(x=w585) -> (x > 0?=w584:bool)
                }
                n268 = Or Array Elements(Boolean array=w582) -> (logical OR=w581:bool)
              }
            }
          }
          frame #5 {
            n269 = case shown="True" w587 {
              tunnel: [TRUE ("T button?") w593] -> w588
              frame False {
              }
              frame True {
                w594 = "EnFlo_Tunnel:Gas Solenoid:Status"
                n270 = Build Array(w594) -> (w597:string[])
                n271 = call "Get_Current_Scan_client.vi"("ADAM Ch Names"=w597) -> ("Numerical Values"=w596:dbl[])  [unwired: 3 out]
                n272 = Index Array(array=w596, index=0) -> (element=w592:dbl)
                n273 = Greater?(x=w592, y=0.5) -> (0:w590:bool)
                n274 = case shown="False" w590 {
                  tunnel: w594 -> [w603 _]
                  tunnel: [w598 TRUE ("T button?")] -> w593
                  frame False {
                    n275 = Format Into String(format string="The \"%s\" ADAM channel is showing that the blue gas button is not on.", w603) -> (resulting string=w601:string)  [unwired: 2 in, 1 out]
                    n276 = Two Button Dialog(message=w601, 1:"Stop" ("F button name (\"Cancel\")"), 2:"Continue" ("T button name (\"OK\")")) -> (T button?=w598:bool)
                  }
                  frame True {
                  }
                }
              }
            }
          }
          frame #6 {
            n277 = case shown="True" w605 {
              frame False {
              }
              frame True {
                n278 = call "Program_Active_Client.vi"("Mode"=enum16{"Program Active", "Traverse Level State"}."Traverse Level State", "Traverse level State"=Traverse_Level_State."Running") -> ()  [unwired: 1 in, 3 out]
              }
            }
          }
        }
      }
      frame "Skip Blank Rows" {
        n279 = stacked-sequence {
          tunnel: w612 -> [w615 w634]
          tunnel: w609 -> [w613 w630]
          frame #0 {
            n280 = Decrement(x=w615) -> (x-1=w614:i32)
            n281 = while {
              tunnel: w613 -> [w625]
              tunnel: w614 -> [w619]
              stop <- w616 continue-if-true
              n282 = local read "Currently on Row"() -> (w621:i32)
              n283 = Increment(x=w621) -> (x+1=w620:i32)
              n284 = Index Array(array=w625, index=w620) -> (element=w624:T6)
              n285 = Less?(x=w620, y=w619) -> (x < y?=w618:bool)
              n286 = Unbundle By Name(w624) -> ("Row Type Selector"=w623:T8)
              n287 = Equal?(x=Multi_run_mode."Blank Row" ("Row Type Selector"), y=w623) -> (x = y?=w617:bool)
              n288 = And(x=w617, y=w618) -> (x .and. y?=w616:bool)
              n289 = case shown="True" w617 {
                tunnel: w620 -> [_ w626]
                frame False {
                }
                frame True {
                  n290 = local write "Currently on Row"(w626) -> ()
                }
              }
            }
          }
          frame #1 {
            n291 = local read "Currently on Row"() -> (w632:i32)
            n292 = Increment(x=w632) -> (x+1=w631:i32)
            n293 = Index Array(array=w630, index=w631) -> (element=w633:T6)
            n294 = Unbundle By Name(w633) -> ("Row Type Selector"=w629:T8)
            n295 = Equal?(x=Multi_run_mode."Turn Off Row Repeating" ("Row Type Selector"), y=w629) -> (x = y?=w627:bool)
            n296 = while {
              shift-right: [w643] -> _
              shift-left: _ -> [w642]
              tunnel: w634 -> [w639]
              tunnel: w632 -> [w643]
              tunnel: w627 -> [w636]
              stop <- TRUE stop-if-true
              n297 = Decrement(x=w639) -> (x-1=w644:i32)
              n298 = Equal?(x=w643, y=w644) -> (x = y?=w637:bool)
              n299 = Not Equal?(x=w643, y=w642) -> (x != y?=w641:bool)
              n300 = Or(x=w636, y=w637) -> (x .or. y?=w635:bool)
              n301 = And(x=w641, y=w635) -> (x .and. y?=w640:bool)
              n302 = case shown="True" w640 {
                tunnel: w639 -> [_ w645]
                frame False {
                }
                frame True {
                  n303 = Initialize Array(timestamp(0 s since 1904-01-01) ("seconds since 1Jan1904"), w645) -> (w647:timestamp[])
                  n304 = global write "Trav_pos_global.vi" "Row completion times"(w647) -> ()
                }
              }
            }
          }
        }
      }
      frame "Which row to execute next" {
        # "last"
        # "Repeat\nRow"
        n305 = local read "Currently on Row"() -> (w648:i32)
        n306 = stacked-sequence {
          seq-local: [_ w677 _] -> [_ _ w714]
          seq-local: [_ w676 _] -> [_ _ w715]
          seq-local: [w657 _ _] -> [_ w675 _]
          seq-local: [_ w672 _] -> [_ _ w708]
          tunnel: [w660 _ _] -> w654
          tunnel: w653 -> [w660 w679 w722]
          tunnel: w652 -> [_ _ w720]
          tunnel: w651 -> [_ w674 w721]
          tunnel: [_ _ w717] -> w650
          tunnel: w649 -> [_ _ w716]
          tunnel: w648 -> [w661 w671 w707]
          frame #0 {
            n307 = Increment(x=w661) -> (x+1=w659:i32)
            n308 = for {
              N: w659 -> [_]
              tunnel: w660 -> [w670] mode=indexing
              shift-right: [w667] -> w657
              shift-left: -1 -> [w664]
              i -> [w665]
              n309 = Unbundle By Name(w670) -> ("Row Type Selector"=w669:T8)
              n310 = Equal?(x=Multi_run_mode."Turn Off Row Repeating" ("Row Type Selector"), y=w669) -> (x = y?=w666:bool)
              n311 = Select(t=w665, s=w666, f=w664) -> (s? t:f=w667:i32)
            }
            n312 = global write "Trav_pos_global.vi" "Paused During Row?"(FALSE ("Paused During Row?")) -> ()
            n313 = global write "Trav_pos_global.vi" "Currently on point"(0 ("Currently on point")) -> ()
          }
          frame #1 {
            n314 = global read "Trav_pos_global.vi" "Row completion times"() -> (w678:timestamp[])
            n315 = global read "Extra_Commands_Global.vi" "Minutes Before Repeating Row"() -> (w673:string)
            n316 = case shown="\"Run VI\"" w674 {
              tunnel: [w680 w681] -> w672
              frame "Check VI only" {
                n317 = global read "Trav_pos_global.vi" "Simulation Time"() -> (w680:timestamp)
              }
              frame "Run VI" {
                n318 = Get Date/Time In Seconds() -> (seconds since 1Jan1904=w681:timestamp)
                n319 = global write "Trav_pos_global.vi" "Simulation Time"(w681) -> ()
              }
            }
            n320 = while {
              tunnel: w679 -> [w692] mode=indexing
              tunnel: w678 -> [w695]
              tunnel: w672 -> [w694]
              tunnel: [w686] -> w677
              tunnel: [w684] -> w676
              tunnel: w675 -> [w683]
              tunnel: w671 -> [w687]
              tunnel: w673 -> [w685]
              i -> [w684]
              stop <- w691 continue-if-true
              n321 = Unbundle By Name(w692) -> ("Extra Commands"=w696:string)
              n322 = call "Extra_Commands.vi"("String to Search"=w696, "Command"=w685) -> ("Numeric Value"=w693:dbl, "Command Found"=w689:bool)  [unwired: 1 in, 3 out]
              n323 = Greater?(x=w684, y=w683) -> (0:w682:bool)
              n324 = And(x=w682, y=w689) -> (x .and. y?=w688:bool)
              n325 = case shown="True" w688 {
                tunnel: w695 -> [_ w702]
                tunnel: w694 -> [_ w703]
                tunnel: w684 -> [_ w701]
                tunnel: w693 -> [_ w699]
                tunnel: [FALSE w698] -> w686
                frame False {
                }
                frame True {
                  n326 = Index Array(array=w702, index=w701) -> (element=w704:timestamp)
                  n327 = Subtract(x=w703, y=w704) -> (x-y=w705:dbl)
                  n328 = Divide(x=w705, y=60.0) -> (x/y=w700:dbl)
                  n329 = Greater?(x=w700, y=w699) -> (0:w698:bool)
                }
              }
              n330 = Less?(x=w684, y=w687) -> (x < y?=w690:bool)
              n331 = Compound Arithmetic op=AND(invert w686, w690) -> (w691:bool)
            }
          }
          frame #2 {
            n332 = Not Equal?(x=w707, y=w715) -> (x != y?=w713:bool)
            n333 = And(x=w714, y=w713) -> (x .and. y?=w712:bool)
            n334 = case shown="True" w712 {
              tunnel: w715 -> [_ w748]
              tunnel: w707 -> [w744 w749]
              tunnel: [w743 w747] -> w718
              tunnel: [w743 w748] -> w709
              tunnel: w720 -> [w746 _]
              tunnel: [w742 TRUE] -> w719
              frame False {
                n335 = Increment(x=w744) -> (x+1=w745:i32)
                n336 = Greater?(x=w746, y=w745) -> (0:w742:bool)
                n337 = Select(t=w745, s=w742, f=w744) -> (s? t:f=w743:i32)
              }
              frame True {
                n338 = Max & Min(x=w749, y=w748) -> (max(x,y)=w747:i32)  [unwired: 1 out]
              }
            }
            n339 = global read "Trav_pos_global.vi" "Row completion times"() -> (w711:timestamp[])
            n340 = case shown="True" w719 {
              tunnel: w709 -> [_ w730]
              tunnel: w722 -> [_ w736]
              tunnel: w721 -> [w724 w728]
              tunnel: w718 -> [_ w734]
              tunnel: [w723 w733] -> w717
              tunnel: w716 -> [_ w733]
              frame False {
                n341 = case shown="\"Run VI\"" w724 {
                  tunnel: [Multi_Run_Case."Show jumped positions" ("Multi Run Case") Multi_Run_Case."Shut down source etc" ("Multi Run Case")] -> w723
                  frame "Check VI only" {
                  }
                  frame "Run VI" {
                  }
                }
              }
              frame True {
                n342 = Index Array(array=w736, index=w730) -> (element=w732:T6)
                n343 = Bundle By Name(cluster=w732, "Row No"=w730) -> (w731:T6)
                n344 = Build Array(w734) -> (w735:i32[])
                n345 = global write "Trav_pos_global.vi" "Meas Setup Number"(0 ("Meas Setup Number")) -> ()
                n346 = property on="Table" class="Arr (strict)"("Index Values"=w735) -> ()  [unwired: 2 in, 2 out]
                n347 = case shown="\"Run VI\"" w728 {
                  selector: w728 -> [_ w738]
                  tunnel: w731 -> [w737 w740]
                  tunnel: [w737 w739] -> w727
                  frame "Check VI only" {
                  }
                  frame "Run VI" {
                    n348 = call "Log_Current_row_to_Execute.vi"("Simulate/Run"=w738, "Start of Multi Run Prog"=FALSE, "Traverse line in"=w740) -> ("Traverse line Out"=w739:T6)  [unwired: 2 in, 4 out]
                  }
                }
                n349 = global write "Trav_pos_global.vi" "Current Row"(w727) -> ()
                "Currently on Row" <- w734
              }
            }
            n350 = Replace Array Subset(array=w711, new element=w708, index=w709) -> (w710:timestamp[])
            n351 = global write "Trav_pos_global.vi" "Row completion times"(w710) -> ()
          }
        }
      }
      frame "Evaluate IF Statement" {
        n352 = global read "Trav_pos_global.vi" "Current Row"() -> (w755:T6)
        n353 = Unbundle By Name(w755) -> ("Extra Commands"=w756:string)
        n354 = global read "Extra_Commands_Global.vi" "If Command"() -> (w759:string)
        n355 = call "Extra_Commands.vi"("String to Search"=w756, "Command"=w759) -> ("String Value"=w758:string, "Command Found"=w752:bool)  [unwired: 1 in, 3 out]
        n356 = And(x=w751, y=w752) -> (x .and. y?=w753:bool)
        n357 = case shown="True" w753 {
          tunnel: w758 -> [_ w769]
          tunnel: [w765 w768] -> w754
          frame False {
            w765 = TRUE  # Execute Row?
          }
          frame True {
            n358 = call "Get_array_values_fr_String.vi"("String Value"=w769) -> ("Numeric Array"=w767:dbl[], "String array"=w766:string[])
            n359 = Index Array(array=w766, index=0 ("Index")) -> (element=w770:string)
            n360 = case shown="\"ADAM Channel Between\"" w770 {
              tunnel: w769 -> [w775 _ _ _]
              tunnel: [w774 w776 w786 TRUE ("Execute Row?")] -> w768
              tunnel: w767 -> [_ w782 w800 _]
              tunnel: w766 -> [_ _ w794 _]
              frame "Time Between" {
                n361 = Get Date/Time In Seconds() -> (seconds since 1Jan1904=w772:timestamp)
                n362 = To Double Precision Float(number=w772) -> (double precision float=w773:dbl)
                n363 = call "If_Time_arguments.vi"("seconds since 1Jan1904"=w773, "String Value"=w775) -> ("Execute Row?"=w774:bool)  [unwired: 2 out]
              }
              frame "Global Value Between" {
                n364 = global read "Extra_Commands_Global.vi" "If command global value"() -> (w777:dbl)
                n365 = Index Array(array=w782, index=1 ("Index")) -> (element=w780:dbl)
                n366 = Index Array(array=w782, index=2 ("Index")) -> (element=w781:dbl)
                n367 = Max & Min(x=w780, y=w781) -> (max(x,y)=w779:dbl, min(x,y)=w778:dbl)
                n368 = In Range and Coerce(upper limit=w779, x=w777, lower limit=w778) -> (In Range?=w776:bool)  [unwired: 1 out]
              }
              frame "ADAM Channel Between" {
                n369 = Index Array(array=w794, index=1 ("Index")) -> (element=w793:string)
                n370 = Build Array(w793) -> (w792:string[])
                n371 = Index Array(array=w800, index=2 ("Index")) -> (element=w798:dbl)
                n372 = Index Array(array=w800, index=3 ("Index")) -> (element=w799:dbl)
                n373 = Max & Min(x=w798, y=w799) -> (max(x,y)=w797:dbl, min(x,y)=w796:dbl)
                n374 = call "Get_Current_Scan_client.vi"("ADAM Ch Names"=w792) -> ("Numerical Values"=w790:dbl[])  [unwired: 3 out]
                n375 = Index Array(array=w790, index=0 ("Index")) -> (element=w789:dbl)
                n376 = In Range and Coerce(upper limit=w797, x=w789, lower limit=w796) -> (In Range?=w787:bool)  [unwired: 1 out]
                n377 = Not A Number/Path/Refnum?(number/path/refnum=w789) -> (NaN/Path/Refnum?=w788:bool)
                n378 = Select(t=TRUE, s=w788, f=w787) -> (s? t:f=w786:bool)
              }
              frame "No Match", Default {
              }
            }
          }
        }
        n379 = Select(t=w762, s=w754, f=Multi_Run_Case."Calculate Row TIme" ("Multi Run Case")) -> (s? t:f=w761:T3)
      }
      frame "Perform Measurement Setup" {
        n380 = global read "Trav_pos_global.vi" "Current Row"() -> (w806:T6)
        n381 = case shown="\"Run VI\"" w805 {
          selector: w805 -> [_ w810]
          tunnel: w806 -> [_ w811]
          frame "Check VI only" {
          }
          frame "Run VI" {
            n382 = stacked-sequence {
              tunnel: w811 -> [w814 _]
              tunnel: w810 -> [w812 _]
              frame #0 {
                n383 = Unbundle By Name(w814) -> ("Extra Commands"=w813:string)
                n384 = call "Pause_for_server_ch_val.vi"("Extra command string"=w813, "Simulate/Run"=w812) -> ()  [unwired: 2 out]
              }
              frame #1 {
                n385 = Get Date/Time In Seconds() -> (seconds since 1Jan1904=w815:timestamp)
                n386 = To Double Precision Float(number=w815) -> (double precision float=w816:dbl)
                n387 = global write "Trav_pos_global.vi" "Start of Row time (Sec)"(w816) -> ()
              }
            }
          }
        }
      }
      frame "Set Measurement Conditions" {
        w822 = TRUE  # Row Completed
        w821 = FALSE  # Row Completed
        n388 = global read "Trav_pos_global.vi" "Current Row"() -> (w819:T6)
        n389 = Unbundle By Name(w819) -> ("Row Type Selector"=w824:T8)
        n390 = case shown="\"Send Message\"" w824 {
          tunnel: [TRUE FALSE TRUE TRUE TRUE TRUE FALSE TRUE FALSE w873 FALSE FALSE FALSE] -> w829
          tunnel: w819 -> [w837 w840 w843 w846 w849 w852 w855 w858 w867 w872 w894 w897 w900]
          tunnel: [w837 w840 w843 w846 w849 w852 w855 w858 w866 w871 w894 w897 w900] -> w825
          tunnel: [w836 w839 w842 w845 w848 w851 w854 w857 w862 w870 w893 w896 w899] -> w823
          tunnel: w822 -> [w836 _ w842 w845 w848 _ _ _ _ w870 w893 w896 w899]
          tunnel: w821 -> [_ w839 _ _ _ w851 w854 w857 w862 _ _ _ _]
          tunnel: w817 -> [_ _ _ _ _ _ _ _ _ w869 _ _ _]
          frame "Move Traverse Only" {
          }
          frame "Check Beam Power" {
          }
          frame "Set Tunnel Speed Only" {
          }
          frame "Set Source Only" {
          }
          frame "Set Measurement Conditions" {
          }
          frame "Single Measurement" {
          }
          frame "Vertical Profile", Default {
          }
          frame "Scanning Valve Measurement" {
          }
          frame "Run VI Named:" {
            n391 = global read "Extra_Commands_Global.vi" "Skip Source Demand"() -> (w865:string)
            n392 = global read "Extra_Commands_Global.vi" "Establish Exp Conditions (s)"() -> (w861:string)
            n393 = Unbundle By Name(w867) -> ("Extra Commands"=w864:string)
            n394 = Concatenate Strings(w861, " = 0" ("Substring"), w865, w864) -> (w863:string)
            n395 = Bundle By Name(cluster=w867, "Extra Commands"=w863) -> (w866:T6)
          }
          frame "Send Message" {
            n396 = stacked-sequence {
              tunnel: [_ _ FALSE] -> w873
              tunnel: w872 -> [w881 w887 w890]
              tunnel: [_ _ w890] -> w871
              tunnel: w869 -> [w874 _ _]
              frame #0 {
                n397 = Unbundle By Name(w881) -> ("Specific Arguments"=w876:string, "Comments"=w877:string, "Filename"=w879:path)
                n398 = Concatenate Strings(w876, w877) -> (w875:string)
                n399 = Build Array(w879) -> (w878:path[])
                n400 = case shown="\"Run VI\"" w874 {
                  tunnel: "Message" ("Error Type") -> [_ w884]
                  tunnel: w875 -> [_ w883]
                  tunnel: w878 -> [_ w882]
                  frame "Check VI only", Default {
                  }
                  frame "Run VI" {
                    n401 = call "Email_Text_Files.vi"("Filenames"=w882, "message"=w883, "subject ([No Subject])"=w884) -> ()
                  }
                }
              }
              frame #1 {
                n402 = Unbundle By Name(w887) -> ("Extra Commands"=w888:string)
                n403 = global read "Extra_Commands_Global.vi" "Establish Exp Conditions (s)"() -> (w889:string)
                n404 = call "Extra_Commands.vi"("String to Search"=w888, "Command"=w889) -> ("Numeric Value"=w885:dbl)  [unwired: 1 in, 4 out]
                n405 = call "Wait_Seconds_with_display.vi"("Message"="In Send Message Row", "Seconds to wait"=w885) -> ()  [unwired: 2 out]
              }
              frame #2 {
              }
            }
          }
          frame "Fall Back to this Row" {
          }
          frame "Turn Off Row Repeating" {
          }
          frame "Blank Row" {
          }
        }
        n406 = case shown="True" w829 {
          tunnel: w825 -> [_ w902]
          tunnel: w817 -> [_ w906]
          tunnel: [Multi_Run_Status."Continue" ("Status") w903] -> w818
          frame False {
          }
          frame True {
            w905 = 1  # Currently on Point
            n407 = call "Program_Active.vi"() -> ()  [unwired: 1 in]
            n408 = call "Set_Measurement_Conditions.vi"("Simulate/Run"=w906, "Currently on Point"=w905, "Traverse line"=w902) -> ("Status Cluster"=w904:T25)  [unwired: 2 out]
            n409 = Unbundle By Name(w904) -> ("Status"=w903:T2)
          }
        }
        n410 = case shown="\"Continue\"" w818 {
          tunnel: [w833 Multi_Run_Case."Calculate Row TIme" ("Multi Run Case")] -> w828
          tunnel: w827 -> [w834 _]
          tunnel: w823 -> [w831 _]
          frame "Continue" {
            n411 = Select(t=Multi_Run_Case."Calculate Row TIme" ("Multi Run Case"), s=w831, f=w834) -> (s? t:f=w833:T3)
          }
          frame "Jump to Next Point", Default {
          }
        }
        n412 = local write "Status"(w818) -> ()
      }
      frame "Execute Row" {
        n413 = global read "Trav_pos_global.vi" "Current Row"() -> (w908:T6)
        n414 = stacked-sequence {
          tunnel: w909 -> [w913 w924 w926]
          tunnel: w908 -> [w914 w921 w925]
          frame #0 {
            n415 = case shown="\"Check VI only\"" w913 {
              selector: w913 -> [w915 _]
              tunnel: w914 -> [w917 _]
              frame "Check VI only" {
                n416 = Unbundle By Name(w917) -> ("Extra Commands"=w918:string, "Row No"=w920:i32, "Meas Setup File"=w916:string)
                n417 = call "Skip_If Sd_Error_Below.vi"("String to Search"=w918, "Simulate/Run"=w915, "Measurement setup Applied?"=TRUE, "Row Number"=w920, "Measurement Setup File"=w916) -> ()  [unwired: 5 out]
              }
              frame "Run VI" {
              }
            }
          }
          frame #1 {
            n418 = call "Execute_Row.vi"("Simulate/Run"=w924, "Traverse line"=w921) -> ("Status"=w923:T2, "Traverse line out"=w922:T6)  [unwired: 2 out]
            n419 = local write "Status"(w923) -> ()
            n420 = global write "Trav_pos_global.vi" "Current Row"(w922) -> ()
          }
          frame #2 {
            w929 = FALSE  # Empty list
            n421 = call "Remember_RD_Folders.vi"("Empty list"=w929) -> ("List of Folders"=w928:path[])  [unwired: 1 in]
            n422 = for {
              tunnel: w925 -> [w934]
              tunnel: w928 -> [w933] mode=indexing
              tunnel: "Muti_Run_Log.xls" ("name or relative path") -> [w931]
              tunnel: w926 -> [w930]
              n423 = Build Path(base path=w933, name or relative path=w931) -> (appended path=w932:path)
              n424 = call "Log_Current_row_to_Execute.vi"("Simulate/Run"=w930, "Start of Multi Run Prog"=FALSE, "Traverse line in"=w934, "Multi Run Log File"=w932) -> ()  [unwired: 1 in, 5 out]
            }
          }
        }
      }
      frame "Calculate Row TIme" {
        n425 = global read "Trav_pos_global.vi" "Paused During Row?"() -> (w940:bool)
        n426 = local read "Status"() -> (w942:T2)
        n427 = global read "Trav_pos_global.vi" "Current Row"() -> (w939:T6)
        n428 = Equal?(x=w942, y=Multi_Run_Status."Continue" ("Status")) -> (x = y?=w941:bool)
        n429 = Compound Arithmetic op=AND(w941, w936, invert w940) -> (w938:bool)
        n430 = case shown="False" w938 {
          tunnel: w939 -> [w955 w966]
          frame False {
            n431 = global read "Trav_pos_global.vi" "Simulation Time"() -> (w956:timestamp)
            n432 = To Double Precision Float(number=w956) -> (double precision float=w950:dbl)
            n433 = call "Calculate_Row_Time.vi"("Row Start Time (Sec Since 1904)"=w950, "Multi Run Row"=w955) -> ("Scalable Time (Sec)"=w953:dbl, "Fixed Time (Sec)"=w951:dbl)
            n434 = call "Overhead_Factor.vi"("Mode"=Overhead."Read Current Overhead") -> ("Current Overhead Factor"=w954:dbl)  [unwired: 3 in]
            n435 = Multiply(x=w953, y=w954) -> (x*y=w952:dbl)
            n436 = Add(x=w951, y=w952) -> (x+y=w947:dbl)
            n437 = Add(x=w950, y=w947) -> (x+y=w949:dbl)
            n438 = global write "Trav_pos_global.vi" "Start of Row time (Sec)"(w947) -> ()
            n439 = To Time Stamp(1:w949) -> (0:w948:timestamp)
            n440 = global write "Trav_pos_global.vi" "Simulation Time"(w948) -> ()
          }
          frame True {
            n441 = global read "Trav_pos_global.vi" "Start of Row time (Sec)"() -> (w964:dbl)
            n442 = Get Date/Time In Seconds() -> (seconds since 1Jan1904=w959:timestamp)
            n443 = To Double Precision Float(number=w959) -> (double precision float=w958:dbl)
            n444 = call "Calculate_Row_Time.vi"("Row Start Time (Sec Since 1904)"=w964, "Multi Run Row"=w966) -> ("Scalable Time (Sec)"=w960:dbl, "Fixed Time (Sec)"=w962:dbl)
            n445 = Subtract(x=w958, y=w964) -> (x-y=w963:dbl)
            n446 = Subtract(x=w963, y=w962) -> (x-y=w961:dbl)
            n447 = call "Overhead_Factor.vi"("Sum of Ideal times (Sec)"=w960, "Sum of Actual times (Sec)"=w961, "Mode"=Overhead."Update total times") -> ()  [unwired: 1 in, 1 out]
          }
        }
      }
      frame "Update time estimate" {
        n448 = global read "Trav_pos_global.vi" "Current Row"() -> (w970:T6)
        n449 = local read "Currently on Row"() -> (w969:i32)
        n450 = Unbundle By Name(w970) -> ("Row No"=w968:i32)
        n451 = Equal?(x=w968, y=w969) -> (x = y?=w967:bool)
        n452 = case shown="\"Run VI\"" w973 {
          tunnel: w976 -> [w979 w1007]
          tunnel: [w984 w1003] -> w975
          tunnel: w972 -> [_ w1009]
          tunnel: [w983 w1008] -> w971
          tunnel: w969 -> [w981 w1002]
          tunnel: w970 -> [w982 w1006]
          tunnel: w967 -> [w980 w1005]
          frame "Check VI only" {
            n453 = global read "Trav_pos_global.vi" "Simulation Time"() -> (w986:timestamp)
            n454 = To Double Precision Float(number=w986) -> (double precision float=w985:dbl)
            n455 = call "Sec_to_date_filename.vi"("seconds"=w985) -> ("Day"=w988:string, "Time"=w987:string)  [unwired: 2 out]
            n456 = Concatenate Strings(w987, "  " ("Substring"), w988) -> (w983:string)
            n457 = case shown="True" w980 {
              tunnel: w981 -> [_ w999]
              tunnel: [w990 w997] -> w984
              tunnel: w983 -> [_ w996]
              tunnel: w982 -> [_ w995]
              tunnel: w979 -> [w990 w991]
              frame False {
              }
              frame True {
                n458 = global read "Trav_pos_global.vi" "Start of Row time (Sec)"() -> (w994:dbl)
                n459 = Divide(x=w994, y=60.0) -> (x/y=w992:dbl)
                n460 = Bundle By Name(cluster=w995, "Completion time"=w996, "Row Duration (mins)"=w992) -> (w998:T6)
                n461 = Replace Array Subset(array=w991, new element=w998, index=w999) -> (w997:T6[])
              }
            }
          }
          frame "Run VI" {
            n462 = case shown="True" w1005 {
              tunnel: w1002 -> [_ w1016]
              tunnel: w1007 -> [w1012 w1015]
              tunnel: w1006 -> [_ w1014]
              tunnel: [w1012 w1013] -> w1004
              frame False {
              }
              frame True {
                n463 = Replace Array Subset(array=w1015, new element=w1014, index=w1016) -> (w1013:T6[])
              }
            }
            n464 = Decrement(x=w1009) -> (x-1=w1011:i32)
            n465 = call "Calc_Remaining_Time.vi"("Currently on Row"=w1002, "Table In"=w1004) -> ("Table Out"=w1003:T6[])  [unwired: 1 out]
            n466 = Index Array(array=w1003, index=w1011) -> (element=w1010:T6)
            n467 = Unbundle By Name(w1010) -> ("Completion time"=w1008:string)
            n468 = call "Program_Active_Client.vi"("Mode"=enum16{"Program Active", "Traverse Level State"}."Traverse Level State", "Traverse level State"=Traverse_Level_State."Running") -> ()  [unwired: 1 in, 3 out]
          }
        }
        "Estimated Completion time" <- w971
        n469 = global write "Trav_pos_global.vi" "Estimated Completion time"(w971) -> ()
      }
      frame "Pause Multi Run Program" {
        n470 = while {
          tunnel: "Pause" -> [w1028]
          tunnel: [w1031] -> w1023
          tunnel: w1022 -> [w1030]
          tunnel: w1020 -> [w1029]
          shift-right: [w1028] -> _
          shift-left: _ -> [w1027]
          stop <- TRUE stop-if-true
          n471 = case shown="True" w1028 {
            selector: w1028 -> [_ w1033]
            tunnel: [w1032 w1037] -> w1031
            tunnel: w1030 -> [w1032 w1035]
            tunnel: w1029 -> [_ w1036]
            tunnel: w1027 -> [_ w1034]
            frame False {
            }
            frame True {
              n472 = stacked-sequence {
                tunnel: w1035 -> [_ _ _ _ w1052]
                tunnel: [_ _ _ _ w1053] -> w1037
                tunnel: w1036 -> [w1039 _ _ _ _]
                tunnel: w1033 -> [_ _ _ w1048 _]
                tunnel: w1034 -> [_ _ _ w1047 _]
                frame #0 {
                  n473 = Quotient & Remainder(x=w1039, y=15) -> (x-y*floor(x/y)=w1038:i32)  [unwired: 1 out]
                  n474 = case shown="0" w1038 {
                    frame 0 {
                      n475 = Current VI's Path() -> (path=w1041:path)
                      n476 = call "Bring_to_front.vi"("path"=w1041) -> ()
                    }
                    frame 1, Default {
                    }
                  }
                }
                frame #1 {
                  n477 = global write "Trav_pos_global.vi" "Paused During Row?"(TRUE ("Paused During Row?")) -> ()
                  "Pause message" <- "Multi Run Program Paused!!!!" ("Pause message")
                }
                frame #2 {
                  n478 = property on="Pause message" class="Str"("Visible"=TRUE) -> ()  [unwired: 2 in, 2 out]
                  n479 = Wait Until Next ms Multiple(millisecond multiple=u32 1500) -> ()  [unwired: 1 out]
                }
                frame #3 {
                  n480 = Compound Arithmetic op=AND(w1048, invert w1047) -> (w1046:bool)
                  n481 = case shown="True" w1046 {
                    frame False {
                    }
                    frame True {
                      n482 = call "Program_Active_Client.vi"("Mode"=enum16{"Program Active", "Traverse Level State"}."Program Active", "Time till next contact (Sec)"=12000.0, "Traverse level State"=Traverse_Level_State."Running") -> ()  [unwired: 3 out]
                    }
                  }
                }
                frame #4 {
                  n483 = property on="Pause message" class="Str"("Visible"=FALSE) -> ()  [unwired: 2 in, 2 out]
                  n484 = Wait Until Next ms Multiple(millisecond multiple=u32 1500) -> ()  [unwired: 1 out]
                  n485 = Decrement(x=w1052) -> (x-1=w1053:T3)
                }
              }
            }
          }
        }
        n486 = call "Overhead_Factor.vi"("Mode"=Overhead."Read Current Overhead") -> ("Current Overhead Factor"=→"Current Overhead Factor":dbl)  [unwired: 3 in]
      }
      frame "Do Another Row?" {
        w1065 = Multi_Run_Status."Terminate Run" ("Status")
        n487 = global read "Preference_global.vi" "Server Comms"() -> (w1060:T26)
        n488 = case shown="\"Server Link Healthy\"" w1060 {
          tunnel: [w1074 TRUE] -> w1059
          frame "Server Link Healthy" {
            n489 = Build Array("EnFlo Lab:Emergency_Stop:Happy") -> (w1077:string[])
            n490 = call "Get_Current_Scan_client.vi"("ADAM Ch Names"=w1077) -> ("Numerical Values"=w1079:dbl[])  [unwired: 1 in, 2 out]
            n491 = Index Array(array=w1079) -> (element=w1075:dbl)  [unwired: 1 in]
            n492 = Not A Number/Path/Refnum?(number/path/refnum=w1075) -> (NaN/Path/Refnum?=w1076:bool)
            n493 = case shown="True" w1076 {
              tunnel: w1075 -> [w1082 _]
              tunnel: [w1080 TRUE] -> w1074
              frame False {
                n494 = Greater?(x=w1082, y=0.5) -> (0:w1080:bool)
              }
              frame True {
              }
            }
          }
          frame "Do Not Link To Server" {
          }
        }
        n495 = case shown="False" "Stop after Repeats" {
          tunnel: w1061 -> [_ w1088]
          frame False {
            n496 = local read "Currently on Row"() -> (w1086:i32)
            n497 = Increment(x=w1086) -> (x+1=→"Last Row Run":i32)
          }
          frame True {
            n498 = Decrement(x=w1088) -> (x-1=w1087:i32)
            n499 = local write "Currently on Row"(w1087) -> ()
          }
        }
        n500 = case shown="True" "stop" {
          tunnel: [w1089 w1090] -> w1066
          tunnel: w1065 -> [_ w1090]
          frame False {
            n501 = local read "Status"() -> (w1089:T2)
          }
          frame True {
            n502 = local write "Status"(w1090) -> ()
          }
        }
        n503 = Not Equal?(x=w1065, y=w1066) -> (x != y?=w1064:bool)
        n504 = case shown="True" w1064 {
          tunnel: [w1091 w1095] -> w1057
          tunnel: w1069 -> [w1092 _]
          tunnel: w1066 -> [_ w1096]
          frame False {
            n505 = case shown="\"Run VI\"" w1092 {
              tunnel: [Multi_Run_Case."Show jumped positions" ("Multi Run Case") Multi_Run_Case."Shut down source etc" ("Multi Run Case")] -> w1091
              frame "Check VI only" {
              }
              frame "Run VI" {
              }
            }
          }
          frame True {
            n506 = case shown="\"Jump To Fall Back\"" w1096 {
              tunnel: [Multi_Run_Case."Skip Blank Rows" ("Multi Run Case") Multi_Run_Case."Find Next Fall Back Row" ("Multi Run Case")] -> w1095
              frame "Continue", Default {
              }
              frame "Jump To Fall Back" {
              }
            }
          }
        }
        n507 = local read "Display Mode"() -> (w1056:T5)
        n508 = case shown="False" w1059 {
          tunnel: [Multi_Run_Case."Shut down source etc" ("Multi Run Case") w1073] -> w1058
          tunnel: w1057 -> [_ w1073]
          frame False {
            n509 = local write "Status"(Multi_Run_Status."Terminate Run" ("Status")) -> ()
          }
          frame True {
          }
        }
        n510 = global write "Route_mapping_global.vi" "Display Mode"(w1056) -> ()
      }
      frame "Find Next Fall Back Row" {
        n511 = local read "Currently on Row"() -> (w1101:i32)
        n512 = Increment(x=w1101) -> (x+1=w1100:i32)
        n513 = Greater?(x=w1099, y=w1100) -> (0:w1107:bool)
        n514 = Index Array(array=w1108, index=w1101) -> (element=w1109:T6)
        n515 = Unbundle By Name(w1109) -> ("Row Type Selector"=w1104:T8)
        n516 = Equal?(x=w1104, y=Multi_run_mode."Fall Back to this Row" ("Mode")) -> (x = y?=w1102:bool)
        n517 = case shown="True" w1107 {
          tunnel: [Multi_Run_Case."Skip Blank Rows" ("Multi Run Case") w1116] -> w1106
          tunnel: w1102 -> [_ w1112]
          tunnel: w1101 -> [_ w1113]
          frame False {
          }
          frame True {
            n518 = case shown="False" w1112 {
              tunnel: w1113 -> [w1118 _]
              frame False {
                n519 = Increment(x=w1118) -> (x+1=w1117:i32)
                n520 = local write "Currently on Row"(w1117) -> ()
              }
              frame True {
              }
            }
            n521 = Select(t=Multi_Run_Case."Skip Blank Rows" ("Multi Run Case"), s=w1112, f=Multi_Run_Case."Find Next Fall Back Row" ("Multi Run Case")) -> (s? t:f=w1116:T3)
          }
        }
      }
      frame "Shut down source etc" {
        n522 = for {
          tunnel: w1137 -> [w1159] mode=indexing
          tunnel: Multi_run_mode."Synchronize With:" ("Mode") -> [w1157]
          tunnel: [w1156] -> w1139 mode=indexing
          n523 = Unbundle By Name(w1159) -> ("Row Type Selector"=w1158:T8)
          n524 = Equal?(x=w1158, y=w1157) -> (x = y?=w1156:bool)
        }
        n525 = call "Program_Active_Client.vi"("Mode"=enum16{"Program Active", "Traverse Level State"}."Traverse Level State", "Traverse level State"=Traverse_Level_State."Complete") -> ()  [unwired: 1 in, 3 out]
        n526 = call "Overhead_Factor.vi"("Mode"=Overhead."Re Scale totals to 3 hrs") -> ()  [unwired: 3 in, 1 out]
        n527 = local read "Status"() -> (w1127:T2)
        n528 = global read "Trav_pos_global.vi" "Source Control?"() -> (w1119:bool)
        n529 = global read "Meas_global.vi" "Start Time of experiment"() -> (w1135:dbl)
        n530 = Equal?(x=w1127, y=Multi_Run_Status."Terminate Run" ("Status")) -> (x = y?=w1125:bool)
        n531 = Or Array Elements(Boolean array=w1139) -> (logical OR=w1128:bool)
        n532 = Compound Arithmetic op=AND(w1128, invert w1125) -> (w1129:bool)
        n533 = Get Date/Time In Seconds() -> (seconds since 1Jan1904=w1120:timestamp)
        n534 = case shown="True" w1129 {
          frame False {
          }
          frame True {
            n535 = global read "Preference_global.vi" "Rig Setup"() -> (w1149:string)
            n536 = Concatenate Strings(w1149, ":Program:Sync") -> (w1151:string)
            n537 = Bundle By Name(cluster=T20 {"Channel Name"="", "New Value"=0.0} ("Update Scan Value Cluster"), "Channel Name"=w1151, "New Value"=1000.0 ("Bundle Element")) -> (w1152:T20)
            n538 = Build Array(w1152) -> (w1154:T20[])
            n539 = call "Update_Current_Value_client.vi"("Update array in"=w1154) -> ()  [unwired: 1 in]
          }
        }
        n540 = case shown="True" w1119 {
          frame False {
          }
          frame True {
            w1147 = u32 1  # Time to hold source OFF (microseconds)
            w1148 = u32 0  # Time to hold source ON (microseconds)
            n541 = call "Set_Source.vi"("Source Status"=Client_Source_Status."Not Using", "Simulate/Run"=User_Specific_mode."Run VI") -> ()  [unwired: 2 in, 6 out]
            n542 = call "Arduino_Timed_Release.vi"("Time to hold source ON (microseconds)"=w1148, "Time to hold source OFF (microseconds)"=w1147, "Number of cycles"=u16 1) -> ()  [unwired: 2 out]
          }
        }
        n543 = To Double Precision Float(number=w1120) -> (double precision float=w1136:dbl)
        n544 = Subtract(x=w1136, y=w1135) -> (x-y=w1134:dbl)
        n545 = Greater?(x=w1134, y=300.0) -> (0:w1131:bool)
        n546 = Not(x=w1131) -> (.not. x?=→"Non Starter":bool)
        n547 = Increment(x=w1123) -> (x+1=w1122:T3)
        n548 = Increment(x=w1122) -> (x+1=w1121:T3)
        n549 = Select(t=w1123, s=w1131, f=w1121) -> (s? t:f=w1132:T3)
      }
      frame "Email results to users" {
        n550 = local read "Currently on Row"() -> (w1165:i32)
        n551 = Increment(x=w1165) -> (x+1=w1160:i32)
        n552 = Split 1D Array(array=w1162, index=w1160) -> (first subarray=w1169:T6[], second subarray=w1168:T6[])
        n553 = Array Size(array=w1168) -> (size(s)=w1170:i32)
        n554 = for {
          tunnel: w1169 -> [w1185] mode=indexing
          shift-right: [w1183] -> w1171
          shift-left: string[] [] -> [w1184]
          n555 = Unbundle By Name(w1185) -> ("Row Type Selector"=w1176:T8, "Filename"=w1182:path, "Comments"=w1181:string)
          n556 = Not Equal?(x=Multi_run_mode."Auto Calibrate" ("Row Type Selector"), y=w1176) -> (x != y?=w1178:bool)
          n557 = Empty String/Path?(string/path=w1182) -> (empty?=w1179:bool)
          n558 = Compound Arithmetic op=AND(w1178, invert w1179) -> (w1177:bool)
          n559 = case shown="True" w1177 {
            tunnel: w1184 -> [w1186 w1194]
            tunnel: [w1186 w1193] -> w1183
            tunnel: w1182 -> [_ w1192]
            tunnel: w1181 -> [_ w1190]
            frame False {
            }
            frame True {
              n560 = Path To String(path=w1192) -> (string=w1191:string)
              n561 = Match Pattern(string=w1190, regular expression=" !!Program added comments") -> (after substring=w1187:string)  [unwired: 4 out]
              n562 = Concatenate Strings(w1191, w1187) -> (w1189:string)
              n563 = Build Array (concatenate)(w1194, w1189) -> (w1193:string[])
            }
          }
        }
        n564 = Equal To 0?(x=w1170) -> (x = 0?=w1161:bool)
        n565 = case shown="False" w1161 {
          tunnel: ["Having completed only some of the requested rows." ("Message") ""] -> w1166
          frame False {
          }
          frame True {
          }
        }
        n566 = call "End_of_run_messages.vi"("Message"=w1166, "Subject"="Multi Run Ended", "Attachments"=w1171) -> ()  [unwired: 1 in]
      }
      frame "Save run efficiency" {
        w1208 = FALSE  # append to file? (new file:F)
        w1207 = FALSE  # advisory dialog? (display:T)
        n567 = call "Get_IP_Number.vi"() -> ("Computer Name"=w1196:string)  [unwired: 1 out]
        n568 = Format Into String(format string="Preferences_%s.xls" ("name or relative path"), w1196) -> (resulting string=w1195:string)  [unwired: 2 in, 1 out]
        n569 = call "Setup_Filepath.vi"("Setup File Type"=Setup_Filetype."General", "Filename in"=w1195) -> ("Filename Out"=w1198:path)  [unwired: 1 out]
        n570 = call "Overhead_Factor.vi"("Mode"=Overhead."Read Current Overhead") -> ("Current Overhead Factor"=w1202:dbl)  [unwired: 3 in]
        n571 = Number To Fractional String(number=w1202, precision (6)=i16 4) -> (F-format string=w1200:string)  [unwired: 2 out]
        n572 = call "Read_Characters_From_File.ph.vi"("file path (dialog if empty)"=w1198) -> ("character string"=w1205:string)  [unwired: 1 in, 7 out]
        n573 = call "Replace_data_in_setup_string.vi"("New data string"=w1200, "Input string"=w1205, "Variable name"="Current Overhead Factor") -> ("Appended string"=w1204:string)
        n574 = call "Write_Characters_To_File.vi"("file path (dialog if empty)"=w1198, "advisory dialog? (display:T)"=w1207, "character string"=w1204, "append to file? (new file:F)"=w1208) -> ()  [unwired: 1 in, 4 out]
      }
      frame "Remove Skipped Commands" {
        n575 = for {
          tunnel: w1214 -> [w1222] mode=indexing
          tunnel: [w1221] -> w1213 mode=indexing
          n576 = Unbundle By Name(w1222) -> ("Comments"=w1220:string)
          n577 = Match Pattern(string=w1220, regular expression=" !!Program added comments") -> (before substring=w1219:string)  [unwired: 4 out]
          n578 = Bundle By Name(cluster=w1222, "Comments"=w1219) -> (w1221:T6)
        }
      }
      frame "Show jumped positions" {
        n579 = global read "Trav_pos_global.vi" "Jumped Positions"() -> (w1225:dbl[][])
        n580 = Array Size(array=w1225) -> (size(s)=w1228:i32[])
        n581 = Index Array(array=w1228, index=0) -> (element=w1224:i32)
        n582 = Greater Than 0?(x=w1224) -> (x > 0?=w1226:bool)
        n583 = case shown="True" w1226 {
          tunnel: w1225 -> [_ w1239]
          tunnel: w1224 -> [_ w1238]
          frame False {
            n584 = Current VI's Path() -> (path=w1233:path)
            n585 = Open VI Reference(vi path=w1233) -> (vi reference=w1234:refnum<vi>, error out=w1235:errorcluster)  [unwired: 1 in, 4 out]
            n586 = property class="VI"(reference=w1234, error in=w1235, "Front Panel Window:Is Frontmost"=TRUE) -> (reference out=w1236:refnum<vi>, error out=w1237:errorcluster)
            n587 = Close Reference(reference=w1236, error in (no error)=w1237) -> ()  [unwired: 1 out]
          }
          frame True {
            n588 = stacked-sequence {
              tunnel: w1239 -> [w1240 w1250]
              tunnel: w1238 -> [w1244 _]
              frame #0 {
                w1245 = TRUE  # Open Front Panel
                w1246 = FALSE  # Crash?
                n589 = global read "Trav_pos_global.vi" "Default Traverse Setup"() -> (w1241:string)
                n590 = Format Into String(format string="There are %d points which cannot be reached", w1244) -> (resulting string=w1242:string)  [unwired: 2 in, 1 out]
                n591 = call "Display_Trav_Views.vi"("Current Probe Position"=w1240, "Traverse Name"=w1241, "Open Front Panel"=w1245, "Error Comments"=w1242, "Crash?"=w1246) -> ()  [unwired: 2 in, 4 out]
              }
              frame #1 {
                n592 = local read "Command filename"() -> (w1254:path)
                n593 = Array To Spreadsheet String(array=w1250, 3:"%.1f" ("format string")) -> (spreadsheet string=w1248:string)  [unwired: 1 out]
                n594 = Strip Path(path=w1254) -> (stripped path=w1253:path)  [unwired: 1 out]
                n595 = Build Path(base path=w1253, name or relative path="Jumped_Positions.xls") -> (appended path=w1251:path)
                n596 = call "Write_File_Simple.vi"("append to file? (new file:F)"=FALSE, "character string"=w1248, "file path"=w1251) -> ()  [unwired: 2 out]
              }
            }
          }
        }
      }
      frame "Save Setup to File" {
        w1274 = FALSE  # Start of Multi Run Prog
        n597 = local read "Command filename"() -> (w1261:path)
        n598 = local read "Status"() -> (w1269:T2)
        n599 = local read "Stop after Repeats"() -> (w1272:bool)
        n600 = local read "Last Row Run"() -> (w1257:i32)
        n601 = local read "stop"() -> (w1273:bool)
        n602 = local read "Non Starter"() -> (w1255:bool)
        n603 = Equal?(x=w1269, y=Multi_Run_Status."Continue" ("Status")) -> (x = y?=w1268:bool)
        n604 = Less?(x=w1267, y=T9."Run Multi Run Prog") -> (x < y?=w1256:bool)
        n605 = Decrement(x=w1257) -> (x-1=w1265:i32)
        n606 = Equal?(x=w1258, y=w1257) -> (x = y?=w1281:bool)
        n607 = Equal To 0?(x=w1257) -> (x = 0?=w1280:bool)
        n608 = Compound Arithmetic op=OR(w1272, w1273, w1268) -> (w1271:bool)
        n609 = Select(t=w1257, s=w1271, f=w1265) -> (s? t:f=w1275:i32)
        n610 = call "Current_Filepath.vi"("Short_Name"="Cmd" ("Data Type"), "Filename in"=w1261, "Data Type"="Commands") -> ("Filename Out"=w1260:path)  [unwired: 1 in, 1 out]
        n611 = Compound Arithmetic op=OR(w1281, w1280, w1256, w1255) -> (w1282:bool)
        n612 = Split 1D Array(array=w1286, index=w1275) -> (second subarray=w1289:T6[])  [unwired: 1 out]
        n613 = local read "Work in Tunnel Coordinates?"() -> (w1264:T1)
        n614 = Path To String(path=w1260) -> (string=w1279:string)
        n615 = local read "Jump Bad Positions"() -> (w1263:bool)
        n616 = case shown="False" w1282 {
          tunnel: w1260 -> [w1298 w1332]
          tunnel: [w1297 w1332] -> w1290
          tunnel: w1289 -> [w1295 _]
          tunnel: [w1294 w1333] -> w1288
          tunnel: w1286 -> [w1296 w1333]
          tunnel: w1264 -> [w1293 _]
          tunnel: w1263 -> [w1292 _]
          frame False {
            n617 = stacked-sequence {
              tunnel: w1298 -> [w1300 w1311 _]
              tunnel: [_ w1304 _] -> w1297
              tunnel: w1296 -> [w1303 _ w1316]
              tunnel: w1295 -> [_ _ w1314]
              tunnel: [_ _ w1313] -> w1294
              tunnel: w1293 -> [w1302 _ _]
              tunnel: w1292 -> [w1301 _ _]
              frame #0 {
                n618 = global write "Trav_pos_global.vi" "Sync to server now"(TRUE) -> ()
                n619 = call "Save_Trav_setup.vi"("Work in Tunnel Coordinates?"=w1302, "Trav Table"=w1303, "Jump Bad Positions"=w1301, "Setup filename"=w1300) -> ()  [unwired: 2 out]
              }
              frame #1 {
                n620 = Strip Path(path=w1311) -> (stripped path=w1312:path, name=w1310:string)
                n621 = call "Add_filename_suffix.vi"("Filename"=w1310) -> ("Original Suffix"=w1307:string, "Base name"=w1309:string)  [unwired: 1 in, 2 out]
                n622 = Concatenate Strings(w1309, "_Rem", w1307) -> (w1306:string)
                n623 = Build Path(base path=w1312, name or relative path=w1306) -> (appended path=w1305:path)
                n624 = call "Find_Unique_Filename.vi"("Path In"=w1305) -> ("Unique Path Out"=w1304:path)  [unwired: 1 in, 1 out]
              }
              frame #2 {
                n625 = global read "Extra_Commands_Global.vi" "Minutes Before Repeating Row"() -> (w1317:string)
                n626 = Index Array(array=w1316, index=0) -> (element=w1319:T6)
                n627 = Initialize Array(w1319, 0 ("dimension size")) -> (w1318:T6[])
                n628 = for {
                  shift-right: [w1322] -> w1315
                  shift-left: w1318 -> [w1324]
                  tunnel: w1317 -> [w1326]
                  tunnel: w1316 -> [w1323] mode=indexing
                  n629 = Unbundle By Name(w1323) -> ("Extra Commands"=w1325:string)
                  n630 = call "Extra_Commands.vi"("String to Search"=w1325, "Command"=w1326) -> ("Command Found"=w1327:bool)  [unwired: 1 in, 4 out]
                  n631 = case shown="True" w1327 {
                    tunnel: w1324 -> [w1328 w1331]
                    tunnel: w1323 -> [_ w1330]
                    tunnel: [w1328 w1329] -> w1322
                    frame False {
                    }
                    frame True {
                      n632 = Build Array (concatenate)(w1331, w1330) -> (w1329:T6[])
                    }
                  }
                }
                n633 = Build Array (concatenate)(w1315, w1314) -> (w1313:T6[])
              }
            }
          }
          frame True {
          }
        }
        n634 = Concatenate Strings("Multi run Prog Ended having the setup filename of :" ("Message"), w1279) -> (w1278:string)
        n635 = call "Log_Current_row_to_Execute.vi"("Simulate/Run"=w1277, "Message"=w1278, "Start of Multi Run Prog"=w1274) -> ()  [unwired: 2 in, 5 out]
        n636 = call "Save_Trav_setup.vi"("Work in Tunnel Coordinates?"=w1264, "Trav Table"=w1288, "Jump Bad Positions"=w1263, "Setup filename"=w1290) -> ("Trav Table Out"=w1287:T6[])  [unwired: 1 out]
        n637 = Select(t=w1287, s=w1282, f=w1286) -> (s? t:f=w1285:T6[])
      }
      frame "End" {
        w1336 = ""
        w1338 = path ""
        w1339 = 0 ("No. of pts.")
        w1334 = nan
        n638 = global write "Trav_pos_global.vi" "Top level setup filename"(w1338) -> ()
        n639 = global write "Trav_pos_global.vi" "Estimated Completion time"("") -> ()
        n640 = global write "Trav_pos_global.vi" "Meas Setup Number"(0 ("Meas Setup Number")) -> ()
        n641 = Build Array(u32 0) -> (w1345:u32[])
        n642 = Current VI's Path() -> (path=w1337:path)
        n643 = property on="Table" class="Arr (strict)"("Index Values"=w1345) -> ()  [unwired: 2 in, 2 out]
        n644 = call "Bring_to_front.vi"("path"=w1337) -> ()
        n645 = global read "Trav_pos_global.vi" "Current Row"() -> (w1344:T6)
        n646 = Bundle By Name(cluster=w1344, "Start X"=w1334, "Start Y"=w1334, "Start Z"=w1334, "End X"=w1334, "End Y"=w1334, "End Z"=w1334, "No. of pts."=w1339, "Spacing"=Spacing."Linear", "Filename"=w1338, "Tunnel Speed"=w1334, "Averaging time (min)"=w1334, "Extra Commands"=w1336, "Specific Arguments"=w1336, "Carrier_1 Q (l/min)"=w1334, "Trace Gas Concentration (%)"=w1334, "Carrier_2 Q (l/min)"=w1334, "Comments"=w1336, "Row No"=w1339, "Row Type Selector"=Multi_run_mode."Blank Row", "Completion time"=w1336, "Meas Setup File"=w1336, "Row Duration (mins)"=w1334, "No. of Valid pts."=w1339) -> (w1343:T6)
        n647 = global write "Trav_pos_global.vi" "Current Row"(w1343) -> ()
      }
    }
    n648 = case shown="True" w10 {
      tunnel: w7 -> [_ w17]
      frame False {
      }
      frame True {
        n649 = local write "Table"(w17) -> ()
      }
    }
    "Multi Run Case" <- w12
  }
